vi "RIRetrieval.vi"(0 "Minimization method":u16(ring)=1 items=["LM method", "Simplex Method"], 1 "Extinction Measured Data":T5={"Extinction"=array122x5[610 elements], "Extinction Uncertainty"=array122x5[610 elements], "Size parameters"=array122x5[610 elements], "Number ofSizes"=5.0, "GeometricCrossSection"=[3.1415926535897934e-10, 3.9760782021995823e-10, 4.908738521234053e-10, 5.939573610693203e-10, 7.068583470577035e-10], "WaveLength"=[359.58929, 360.1004, 360.61145, 361.12241, 361.63336, 362.1442, 362.65503, 363.16577, 363.67648, 364.18713, 364.69769, 365.20825, 365.71872, 366.22913, 366.7395, 367.24979, 367.76004, 368.27023, 368.78036, 369.29047, 369.80051, 370.31049, 370.8204, 371.33026, 371.84009, 372.34985, 372.85956, 373.3692, 373.87881, 374.38834, 374.89786, 375.40729, 375.91669, 376.42599, 376.9353, 377.44452, 377.9537, 378.46283, 378.97192, 379.48093, 379.9899, 380.49881, 381.00769, 381.51651, 382.02527, 382.534, 383.04266, 383.55127, 384.05984, 384.56836, 385.07681, 385.58521, 386.09357, 386.6019, 387.11017, 387.61838, 388.12653, 388.63467, 389.14273, 389.65076, 390.15872, 389.65076, 390.15872, 390.66663, 391.17453, 391.68234, 392.19012, 392.69785, 393.20554, 393.71317, 394.22076, 394.7283, 395.23578, 395.74326, 396.25064, 396.758, 397.26532, 397.77258, 398.27979, 398.78696, 399.29407, 399.80115, 400.30817, 400.81516, 401.32211, 401.82901, 402.33585, 402.84265, 403.34943, 403.85614, 404.36282, 404.86945, 405.37604, 405.88257, 406.38907, 406.89554, 407.40195, 407.90833, 408.41464, 408.92093, 409.42715, 409.93335, 410.43951, 410.94562, 411.45169, 411.95773, 412.46371, 412.96964, 413.47556, 413.98141, 414.48724, 414.99301, 415.49875, 416.00446, 416.5101, 417.01572, 417.5213, 418.02682, 418.53235, 419.03778, 419.54321, 420.04858], "Sizes"=[200.0, 225.0, 250.0, 275.0, 300.0], "Concentration (#/cc)"=[]}, 2 "Starting Guess -Real":dbl=1.5, 3 "Approximate Errors":bool, 5 "Graph Refs":T4, 9 "Particle Distribution Data":T6={"SMPS Sizes"=[121.9, 126.3, 131.0, 135.8, 140.7, 145.9, 151.2, 156.8, 162.5, 168.5, 174.7, 181.1, 187.7, 194.6, 201.7, 209.1, 216.7, 224.7, 232.9, 241.4, 250.3, 259.5, 269.0, 278.8, 289.0, 299.6, 310.6, 322.0, 333.8, 346.0, 358.7, 371.8, 385.4, 399.5, 414.2, 429.4, 445.1, 461.4, 478.3, 495.8, 514.0, 532.8, 552.3], "Concentration"=[[0.0, 0.0, 0.0, 0.0, 0.0, 0.0, 0.0, 0.0, 0.0, 0.000594222, 0.0067148, 0.0325883, 0.0950329, 0.181348, 0.216099, 0.185692, 0.101524, 0.0383134, 0.00909043, 0.000780919, 0.0, 0.0, 0.000216077, 0.00198783, 0.0080372, 0.0204479, 0.0283157, 0.0335331, 0.022157, 0.0123005, 0.00284358, 0.000773561, 0.000252233, 0.000229051, 0.000520001, 0.000225684, 0.000138298, 0.000244182, 0.0, 0.0, 0.0, 0.0, 0.0], [0.0, 0.0, 0.0, 0.0, 0.0, 0.0, 0.0, 0.0, 0.0, 0.0, 0.0, 0.0, 0.000816489, 0.00845349, 0.0408459, 0.112602, 0.207837, 0.230678, 0.191195, 0.115028, 0.0385312, 0.00775818, 0.000694285, 0.0, 0.0, 5.45e-05, 0.000573695, 0.00252084, 0.00630844, 0.00962652, 0.0109084, 0.0108076, 0.0029388, 0.00150807, 0.000290999, 2.27e-05, 0.0, 0.0, 0.0, 0.0, 0.0, 0.0, 0.0], [0.0, 0.0, 0.0, 0.0, 0.0, 0.0, 0.0, 0.0, 0.0, 0.0, 0.0, 0.0, 0.0, 0.0, 0.0, 0.0010312, 0.010922, 0.0510087, 0.131879, 0.225192, 0.246535, 0.18825, 0.0982208, 0.0303467, 0.00671228, 0.000607538, 1.36e-05, 0.0, 0.0, 7.85e-05, 0.000394547, 0.00155356, 0.00182002, 0.00285395, 0.00143116, 0.000779854, 0.000340487, 0.0, 0.0, 0.0, 0.0, 0.0, 5.83e-05], [0.0, 0.0, 0.0, 0.0, 0.0, 0.0, 0.0, 0.0, 0.0, 0.0, 0.0, 0.0, 0.0, 0.0, 0.0, 0.0, 0.0, 0.0, 0.00139618, 0.0150043, 0.0584558, 0.144869, 0.242414, 0.233752, 0.174403, 0.0932754, 0.0278801, 0.00466978, 0.000461, 1.86e-05, 0.0, 0.0, 1.87e-05, 0.000141669, 0.000338039, 0.000948904, 0.00124014, 0.000405092, 0.0, 0.000308013, 0.0, 0.0, 0.0], [0.0, 0.0, 0.0, 0.0, 0.0, 0.0, 0.0, 0.0, 0.0, 0.0, 0.0, 0.0, 0.0, 0.0, 0.0, 0.0, 0.0, 0.0, 0.0, 0.0, 0.001984, 0.0181243, 0.0738336, 0.168822, 0.26219, 0.229236, 0.15382, 0.0682415, 0.0199068, 0.0034375, 0.000356967, 1.85e-05, 0.0, 0.0, 7.2e-06, 2.06e-05, 0.0, 0.0, 0.0, 0.0, 0.0, 0.0, 0.0]], "Double Charge Correction Flag"=TRUE}, 11 "Calculate Errors":bool=TRUE, 12 "Restrict to Positive Imaginary Part":bool=TRUE, 13 "Starting Guess - Imag":dbl=0.1, 14 "General Data for RI Retrieval VI":T3={"Min WaveLength Index"=0, "Max WaveLength Index"=121, "Extinction Factor"=FALSE, "Size Parameter Factor"=FALSE, "Size Paramter Offset"=FALSE, "Extinction Factor"=1.0, "Diameter Factor"=1.0, "Diameter Offset"=0.0, "ExtinctionOrAbsorptionOrScattering"=0} {"ExtinctionOrAbsorptionOrScattering" scale=0.0..2.0; "Max WaveLength Index" max=200 step=1; "Min WaveLength Index" max=200 step=1}) -> (4 "Real Part vs wavelength":cluster{dbl[], dbl[]}[](graph)=[{[359.58929, 360.1004, 360.61145, 361.12241, 361.63336, 362.1442, 362.65503, 363.16577, 363.67648, 364.18713, 364.69769, 365.20825, 365.71872, 366.22913, 366.7395, 367.24979, 367.76004, 368.27023, 368.78036, 369.29047, 369.80051, 370.31049, 370.8204, 371.33026, 371.84009, 372.34985, 372.85956, 373.3692, 373.87881, 374.38834, 374.89786, 375.40729, 375.91669, 376.42599, 376.9353, 377.44452, 377.9537, 378.46283, 378.97192, 379.48093, 379.9899, 380.49881, 381.00769, 381.51651, 382.02527, 382.534, 383.04266, 383.55127, 384.05984, 384.56836, 385.07681, 385.58521, 386.09357, 386.6019, 387.11017, 387.61838, 388.12653, 388.63467, 389.14273, 389.65076, 390.15872, 389.65076, 390.15872, 390.66663, 391.17453, 391.68234, 392.19012, 392.69785, 393.20554, 393.71317, 394.22076, 394.7283, 395.23578, 395.74326, 396.25064, 396.758, 397.26532, 397.77258, 398.27979, 398.78696, 399.29407, 399.80115, 400.30817, 400.81516, 401.32211, 401.82901, 402.33585, 402.84265, 403.34943, 403.85614, 404.36282, 404.86945, 405.37604, 405.88257, 406.38907, 406.89554, 407.40195, 407.90833, 408.41464, 408.92093, 409.42715, 409.93335, 410.43951, 410.94562, 411.45169, 411.95773, 412.46371, 412.96964, 413.47556, 413.98141, 414.48724, 414.99301, 415.49875, 416.00446, 416.5101, 417.01572, 417.5213, 418.02682, 418.53235, 419.03778, 419.54321, 420.04858], [1.5396270532046785, 1.538727395001552, 1.534821145001552, 1.5406825036441298, 1.5415669030581922, 1.5455036706363172, 1.5466480798160047, 1.5476615685855357, 1.5472341699038954, 1.5489252824222053, 1.549121510449548, 1.5458964127932977, 1.5447889298831412, 1.5456751603518915, 1.5450364274417363, 1.5443976945315812, 1.5424206728373981, 1.541581134263179, 1.5454557222758747, 1.5423593325053675, 1.537313327256344, 1.5345896334086881, 1.5407291597758752, 1.541564731064938, 1.538654727402829, 1.5370564073955049, 1.5407485765849556, 1.5394119734202825, 1.5341312117015322, 1.536965684357782, 1.5317178816234067, 1.5287030500804377, 1.5274973005687187, 1.5339043898021174, 1.5331876844798522, 1.5293449682628117, 1.5360365600024661, 1.5362565917407474, 1.5274009246264897, 1.5331344623004397, 1.5305994052325689, 1.5268769473468278, 1.5300680369769548, 1.515133306447169, 1.5320916194354501, 1.5417069930468976, 1.537891418400902, 1.5267598266040272, 1.5311928100024632, 1.5343562621509004, 1.5248573607837126, 1.5298715514575405, 1.5194143981372292, 1.521543304387229, 1.5345590919886996, 1.5370029396449496, 1.5382092995082304, 1.5201217598353787, 1.533493494454519, 1.5250244087611615, 1.528523096505302, 1.5305934090053022, 1.5374183601771767, 1.523488001290457, 1.51958495563616, 1.5280126900111597, 1.5125830025111582, 1.5290344185267832, 1.5172637886439704, 1.5226925987635989, 1.5252196068202393, 1.5269847435389892, 1.5132711822425255, 1.5168063384925254, 1.5125790435706503, 1.5172769195472116, 1.5246480590735807, 1.5129183012877858, 1.517646694842472, 1.5133032042418861, 1.5151971251403236, 1.5191888243590723, 1.5131286436950102, 1.5062460143004799, 1.5115656859313376, 1.5106379515563368, 1.512958508196962, 1.511806774798524, 1.5120249754821184, 1.5104307372008678, 1.5129768378173223, 1.5112502867614142, 1.5110824400817269, 1.5072253233825075, 1.502771015826355, 1.5042590529357298, 1.502026997271666, 1.497705746356139, 1.4951637179290151, 1.496234217349181, 1.492047072116026, 1.4983118111525868, 1.4949415547286367, 1.4929246861373284, 1.4926866275702815, 1.490306308928619, 1.4843443567191468, 1.4885330349837649, 1.493107185426842, 1.4893548203145373, 1.4812372971211785, 1.4947460747395862, 1.4976160240804064, 1.4870664024983753, 1.4926434076463098, 1.4957490176593176, 1.4934942263995516, 1.4954207820330967, 1.4921062869464272, 1.493986455861222, 1.4937534350787511, 1.4779602021609655]}, {[359.58929, 359.58929, 359.58929, 360.1004, 360.1004, 360.1004, 360.61145, 360.61145, 360.61145, 361.12241, 361.12241, 361.12241, 361.63336, 361.63336, 361.63336, 362.1442, 362.1442, 362.1442, 362.65503, 362.65503, 362.65503, 363.16577, 363.16577, 363.16577, 363.67648, 363.67648, 363.67648, 364.18713, 364.18713, 364.18713, 364.69769, 364.69769, 364.69769, 365.20825, 365.20825, 365.20825, 365.71872, 365.71872, 365.71872, 366.22913, 366.22913, 366.22913, 366.7395, 366.7395, 366.7395, 367.24979, 367.24979, 367.24979, 367.76004, 367.76004, 367.76004, 368.27023, 368.27023, 368.27023, 368.78036, 368.78036, 368.78036, 369.29047, 369.29047, 369.29047, 369.80051, 369.80051, 369.80051, 370.31049, 370.31049, 370.31049, 370.8204, 370.8204, 370.8204, 371.33026, 371.33026, 371.33026, 371.84009, 371.84009, 371.84009, 372.34985, 372.34985, 372.34985, 372.85956, 372.85956, 372.85956, 373.3692, 373.3692, 373.3692, 373.87881, 373.87881, 373.87881, 374.38834, 374.38834, 374.38834, 374.89786, 374.89786, 374.89786, 375.40729, 375.40729, 375.40729, 375.91669, 375.91669, 375.91669, 376.42599, 376.42599, 376.42599, 376.9353, 376.9353, 376.9353, 377.44452, 377.44452, 377.44452, 377.9537, 377.9537, 377.9537, 378.46283, 378.46283, 378.46283, 378.97192, 378.97192, 378.97192, 379.48093, 379.48093, 379.48093, 379.9899, 379.9899, 379.9899, 380.49881, 380.49881, 380.49881, 381.00769, 381.00769, 381.00769, 381.51651, 381.51651, 381.51651, 382.02527, 382.02527, 382.02527, 382.534, 382.534, 382.534, 383.04266, 383.04266, 383.04266, 383.55127, 383.55127, 383.55127, 384.05984, 384.05984, 384.05984, 384.56836, 384.56836, 384.56836, 385.07681, 385.07681, 385.07681, 385.58521, 385.58521, 385.58521, 386.09357, 386.09357, 386.09357, 386.6019, 386.6019, 386.6019, 387.11017, 387.11017, 387.11017, 387.61838, 387.61838, 387.61838, 388.12653, 388.12653, 388.12653, 388.63467, 388.63467, 388.63467, 389.14273, 389.14273, 389.14273, 389.65076, 389.65076, 389.65076, 390.15872, 390.15872, 390.15872, 389.65076, 389.65076, 389.65076, 390.15872, 390.15872, 390.15872, 390.66663, 390.66663, 390.66663, 391.17453, 391.17453, 391.17453, 391.68234, 391.68234, 391.68234, 392.19012, 392.19012, 392.19012, 392.69785, 392.69785, 392.69785, 393.20554, 393.20554, 393.20554, 393.71317, 393.71317, 393.71317, 394.22076, 394.22076, 394.22076, 394.7283, 394.7283, 394.7283, 395.23578, 395.23578, 395.23578, 395.74326, 395.74326, 395.74326, 396.25064, 396.25064, 396.25064, 396.758, 396.758, 396.758, 397.26532, 397.26532, 397.26532, 397.77258, 397.77258, 397.77258, 398.27979, 398.27979, 398.27979, 398.78696, 398.78696, 398.78696, 399.29407, 399.29407, 399.29407, 399.80115, 399.80115, 399.80115, 400.30817, 400.30817, 400.30817, 400.81516, 400.81516, 400.81516, 401.32211, 401.32211, 401.32211, 401.82901, 401.82901, 401.82901, 402.33585, 402.33585, 402.33585, 402.84265, 402.84265, 402.84265, 403.34943, 403.34943, 403.34943, 403.85614, 403.85614, 403.85614, 404.36282, 404.36282, 404.36282, 404.86945, 404.86945, 404.86945, 405.37604, 405.37604, 405.37604, 405.88257, 405.88257, 405.88257, 406.38907, 406.38907, 406.38907, 406.89554, 406.89554, 406.89554, 407.40195, 407.40195, 407.40195, 407.90833, 407.90833, 407.90833, 408.41464, 408.41464, 408.41464, 408.92093, 408.92093, 408.92093, 409.42715, 409.42715, 409.42715, 409.93335, 409.93335, 409.93335, 410.43951, 410.43951, 410.43951, 410.94562, 410.94562, 410.94562, 411.45169, 411.45169, 411.45169, 411.95773, 411.95773, 411.95773, 412.46371, 412.46371, 412.46371, 412.96964, 412.96964, 412.96964, 413.47556, 413.47556, 413.47556, 413.98141, 413.98141, 413.98141, 414.48724, 414.48724, 414.48724, 414.99301, 414.99301, 414.99301, 415.49875, 415.49875, 415.49875, 416.00446, 416.00446, 416.00446, 416.5101, 416.5101, 416.5101, 417.01572, 417.01572, 417.01572, 417.5213, 417.5213, 417.5213, 418.02682, 418.02682, 418.02682, 418.53235, 418.53235, 418.53235, 419.03778, 419.03778, 419.03778, 419.54321, 419.54321, 419.54321, 420.04858, 420.04858, 420.04858], [nan, 1.5396270532046785, 1.5396270532046785, nan, 1.538727395001552, 1.538727395001552, nan, 1.534821145001552, 1.534821145001552, nan, 1.5406825036441298, 1.5406825036441298, nan, 1.5415669030581922, 1.5415669030581922, nan, 1.5455036706363172, 1.5455036706363172, nan, 1.5466480798160047, 1.5466480798160047, nan, 1.5476615685855357, 1.5476615685855357, nan, 1.5472341699038954, 1.5472341699038954, nan, 1.5489252824222053, 1.5489252824222053, nan, 1.549121510449548, 1.549121510449548, nan, 1.5458964127932977, 1.5458964127932977, nan, 1.5447889298831412, 1.5447889298831412, nan, 1.5456751603518915, 1.5456751603518915, nan, 1.5450364274417363, 1.5450364274417363, nan, 1.5443976945315812, 1.5443976945315812, nan, 1.5424206728373981, 1.5424206728373981, nan, 1.541581134263179, 1.541581134263179, nan, 1.5454557222758747, 1.5454557222758747, nan, 1.5423593325053675, 1.5423593325053675, nan, 1.537313327256344, 1.537313327256344, nan, 1.5345896334086881, 1.5345896334086881, nan, 1.5407291597758752, 1.5407291597758752, nan, 1.541564731064938, 1.541564731064938, nan, 1.538654727402829, 1.538654727402829, nan, 1.5370564073955049, 1.5370564073955049, nan, 1.5407485765849556, 1.5407485765849556, nan, 1.5394119734202825, 1.5394119734202825, nan, 1.5341312117015322, 1.5341312117015322, nan, 1.536965684357782, 1.536965684357782, nan, 1.5317178816234067, 1.5317178816234067, nan, 1.5287030500804377, 1.5287030500804377, nan, 1.5274973005687187, 1.5274973005687187, nan, 1.5339043898021174, 1.5339043898021174, nan, 1.5331876844798522, 1.5331876844798522, nan, 1.5293449682628117, 1.5293449682628117, nan, 1.5360365600024661, 1.5360365600024661, nan, 1.5362565917407474, 1.5362565917407474, nan, 1.5274009246264897, 1.5274009246264897, nan, 1.5331344623004397, 1.5331344623004397, nan, 1.5305994052325689, 1.5305994052325689, nan, 1.5268769473468278, 1.5268769473468278, nan, 1.5300680369769548, 1.5300680369769548, nan, 1.515133306447169, 1.515133306447169, nan, 1.5320916194354501, 1.5320916194354501, nan, 1.5417069930468976, 1.5417069930468976, nan, 1.537891418400902, 1.537891418400902, nan, 1.5267598266040272, 1.5267598266040272, nan, 1.5311928100024632, 1.5311928100024632, nan, 1.5343562621509004, 1.5343562621509004, nan, 1.5248573607837126, 1.5248573607837126, nan, 1.5298715514575405, 1.5298715514575405, nan, 1.5194143981372292, 1.5194143981372292, nan, 1.521543304387229, 1.521543304387229, nan, 1.5345590919886996, 1.5345590919886996, nan, 1.5370029396449496, 1.5370029396449496, nan, 1.5382092995082304, 1.5382092995082304, nan, 1.5201217598353787, 1.5201217598353787, nan, 1.533493494454519, 1.533493494454519, nan, 1.5250244087611615, 1.5250244087611615, nan, 1.528523096505302, 1.528523096505302, nan, 1.5305934090053022, 1.5305934090053022, nan, 1.5374183601771767, 1.5374183601771767, nan, 1.523488001290457, 1.523488001290457, nan, 1.51958495563616, 1.51958495563616, nan, 1.5280126900111597, 1.5280126900111597, nan, 1.5125830025111582, 1.5125830025111582, nan, 1.5290344185267832, 1.5290344185267832, nan, 1.5172637886439704, 1.5172637886439704, nan, 1.5226925987635989, 1.5226925987635989, nan, 1.5252196068202393, 1.5252196068202393, nan, 1.5269847435389892, 1.5269847435389892, nan, 1.5132711822425255, 1.5132711822425255, nan, 1.5168063384925254, 1.5168063384925254, nan, 1.5125790435706503, 1.5125790435706503, nan, 1.5172769195472116, 1.5172769195472116, nan, 1.5246480590735807, 1.5246480590735807, nan, 1.5129183012877858, 1.5129183012877858, nan, 1.517646694842472, 1.517646694842472, nan, 1.5133032042418861, 1.5133032042418861, nan, 1.5151971251403236, 1.5151971251403236, nan, 1.5191888243590723, 1.5191888243590723, nan, 1.5131286436950102, 1.5131286436950102, nan, 1.5062460143004799, 1.5062460143004799, nan, 1.5115656859313376, 1.5115656859313376, nan, 1.5106379515563368, 1.5106379515563368, nan, 1.512958508196962, 1.512958508196962, nan, 1.511806774798524, 1.511806774798524, nan, 1.5120249754821184, 1.5120249754821184, nan, 1.5104307372008678, 1.5104307372008678, nan, 1.5129768378173223, 1.5129768378173223, nan, 1.5112502867614142, 1.5112502867614142, nan, 1.5110824400817269, 1.5110824400817269, nan, 1.5072253233825075, 1.5072253233825075, nan, 1.502771015826355, 1.502771015826355, nan, 1.5042590529357298, 1.5042590529357298, nan, 1.502026997271666, 1.502026997271666, nan, 1.497705746356139, 1.497705746356139, nan, 1.4951637179290151, 1.4951637179290151, nan, 1.496234217349181, 1.496234217349181, nan, 1.492047072116026, 1.492047072116026, nan, 1.4983118111525868, 1.4983118111525868, nan, 1.4949415547286367, 1.4949415547286367, nan, 1.4929246861373284, 1.4929246861373284, nan, 1.4926866275702815, 1.4926866275702815, nan, 1.490306308928619, 1.490306308928619, nan, 1.4843443567191468, 1.4843443567191468, nan, 1.4885330349837649, 1.4885330349837649, nan, 1.493107185426842, 1.493107185426842, nan, 1.4893548203145373, 1.4893548203145373, nan, 1.4812372971211785, 1.4812372971211785, nan, 1.4947460747395862, 1.4947460747395862, nan, 1.4976160240804064, 1.4976160240804064, nan, 1.4870664024983753, 1.4870664024983753, nan, 1.4926434076463098, 1.4926434076463098, nan, 1.4957490176593176, 1.4957490176593176, nan, 1.4934942263995516, 1.4934942263995516, nan, 1.4954207820330967, 1.4954207820330967, nan, 1.4921062869464272, 1.4921062869464272, nan, 1.493986455861222, 1.493986455861222, nan, 1.4937534350787511, 1.4937534350787511, nan, 1.4779602021609655, 1.4779602021609655]}, {[359.58929, 360.1004, 360.61145, 361.12241, 361.63336, 362.1442, 362.65503, 363.16577, 363.67648, 364.18713, 364.69769, 365.20825, 365.71872, 366.22913, 366.7395, 367.24979, 367.76004, 368.27023, 368.78036, 369.29047, 369.80051, 370.31049, 370.8204, 371.33026, 371.84009, 372.34985, 372.85956, 373.3692, 373.87881, 374.38834, 374.89786, 375.40729, 375.91669, 376.42599, 376.9353, 377.44452, 377.9537, 378.46283, 378.97192, 379.48093, 379.9899, 380.49881, 381.00769, 381.51651, 382.02527, 382.534, 383.04266, 383.55127, 384.05984, 384.56836, 385.07681, 385.58521, 386.09357, 386.6019, 387.11017, 387.61838, 388.12653, 388.63467, 389.14273, 389.65076, 390.15872, 389.65076, 390.15872, 390.66663, 391.17453, 391.68234, 392.19012, 392.69785, 393.20554, 393.71317, 394.22076, 394.7283, 395.23578, 395.74326, 396.25064, 396.758, 397.26532, 397.77258, 398.27979, 398.78696, 399.29407, 399.80115, 400.30817, 400.81516, 401.32211, 401.82901, 402.33585, 402.84265, 403.34943, 403.85614, 404.36282, 404.86945, 405.37604, 405.88257, 406.38907, 406.89554, 407.40195, 407.90833, 408.41464, 408.92093, 409.42715, 409.93335, 410.43951, 410.94562, 411.45169, 411.95773, 412.46371, 412.96964, 413.47556, 413.98141, 414.48724, 414.99301, 415.49875, 416.00446, 416.5101, 417.01572, 417.5213, 418.02682, 418.53235, 419.03778, 419.54321, 420.04858], [1.5396270532046785, 1.538727395001552, 1.534821145001552, 1.5406825036441298, 1.5415669030581922, 1.5455036706363172, 1.5466480798160047, 1.5476615685855357, 1.5472341699038954, 1.5489252824222053, 1.549121510449548, 1.5458964127932977, 1.5447889298831412, 1.5456751603518915, 1.5450364274417363, 1.5443976945315812, 1.5424206728373981, 1.541581134263179, 1.5454557222758747, 1.5423593325053675, 1.537313327256344, 1.5345896334086881, 1.5407291597758752, 1.541564731064938, 1.538654727402829, 1.5370564073955049, 1.5407485765849556, 1.5394119734202825, 1.5341312117015322, 1.536965684357782, 1.5317178816234067, 1.5287030500804377, 1.5274973005687187, 1.5339043898021174, 1.5331876844798522, 1.5293449682628117, 1.5360365600024661, 1.5362565917407474, 1.5274009246264897, 1.5331344623004397, 1.5305994052325689, 1.5268769473468278, 1.5300680369769548, 1.515133306447169, 1.5320916194354501, 1.5417069930468976, 1.537891418400902, 1.5267598266040272, 1.5311928100024632, 1.5343562621509004, 1.5248573607837126, 1.5298715514575405, 1.5194143981372292, 1.521543304387229, 1.5345590919886996, 1.5370029396449496, 1.5382092995082304, 1.5201217598353787, 1.533493494454519, 1.5250244087611615, 1.528523096505302, 1.5305934090053022, 1.5374183601771767, 1.523488001290457, 1.51958495563616, 1.5280126900111597, 1.5125830025111582, 1.5290344185267832, 1.5172637886439704, 1.5226925987635989, 1.5252196068202393, 1.5269847435389892, 1.5132711822425255, 1.5168063384925254, 1.5125790435706503, 1.5172769195472116, 1.5246480590735807, 1.5129183012877858, 1.517646694842472, 1.5133032042418861, 1.5151971251403236, 1.5191888243590723, 1.5131286436950102, 1.5062460143004799, 1.5115656859313376, 1.5106379515563368, 1.512958508196962, 1.511806774798524, 1.5120249754821184, 1.5104307372008678, 1.5129768378173223, 1.5112502867614142, 1.5110824400817269, 1.5072253233825075, 1.502771015826355, 1.5042590529357298, 1.502026997271666, 1.497705746356139, 1.4951637179290151, 1.496234217349181, 1.492047072116026, 1.4983118111525868, 1.4949415547286367, 1.4929246861373284, 1.4926866275702815, 1.490306308928619, 1.4843443567191468, 1.4885330349837649, 1.493107185426842, 1.4893548203145373, 1.4812372971211785, 1.4947460747395862, 1.4976160240804064, 1.4870664024983753, 1.4926434076463098, 1.4957490176593176, 1.4934942263995516, 1.4954207820330967, 1.4921062869464272, 1.493986455861222, 1.4937534350787511, 1.4779602021609655]}], 6 "RI results":T2={"Real RI"=[1.5396270532046785, 1.538727395001552, 1.534821145001552, 1.5406825036441298, 1.5415669030581922, 1.5455036706363172, 1.5466480798160047, 1.5476615685855357, 1.5472341699038954, 1.5489252824222053, 1.549121510449548, 1.5458964127932977, 1.5447889298831412, 1.5456751603518915, 1.5450364274417363, 1.5443976945315812, 1.5424206728373981, 1.541581134263179, 1.5454557222758747, 1.5423593325053675, 1.537313327256344, 1.5345896334086881, 1.5407291597758752, 1.541564731064938, 1.538654727402829, 1.5370564073955049, 1.5407485765849556, 1.5394119734202825, 1.5341312117015322, 1.536965684357782, 1.5317178816234067, 1.5287030500804377, 1.5274973005687187, 1.5339043898021174, 1.5331876844798522, 1.5293449682628117, 1.5360365600024661, 1.5362565917407474, 1.5274009246264897, 1.5331344623004397, 1.5305994052325689, 1.5268769473468278, 1.5300680369769548, 1.515133306447169, 1.5320916194354501, 1.5417069930468976, 1.537891418400902, 1.5267598266040272, 1.5311928100024632, 1.5343562621509004, 1.5248573607837126, 1.5298715514575405, 1.5194143981372292, 1.521543304387229, 1.5345590919886996, 1.5370029396449496, 1.5382092995082304, 1.5201217598353787, 1.533493494454519, 1.5250244087611615, 1.528523096505302, 1.5305934090053022, 1.5374183601771767, 1.523488001290457, 1.51958495563616, 1.5280126900111597, 1.5125830025111582, 1.5290344185267832, 1.5172637886439704, 1.5226925987635989, 1.5252196068202393, 1.5269847435389892, 1.5132711822425255, 1.5168063384925254, 1.5125790435706503, 1.5172769195472116, 1.5246480590735807, 1.5129183012877858, 1.517646694842472, 1.5133032042418861, 1.5151971251403236, 1.5191888243590723, 1.5131286436950102, 1.5062460143004799, 1.5115656859313376, 1.5106379515563368, 1.512958508196962, 1.511806774798524, 1.5120249754821184, 1.5104307372008678, 1.5129768378173223, 1.5112502867614142, 1.5110824400817269, 1.5072253233825075, 1.502771015826355, 1.5042590529357298, 1.502026997271666, 1.497705746356139, 1.4951637179290151, 1.496234217349181, 1.492047072116026, 1.4983118111525868, 1.4949415547286367, 1.4929246861373284, 1.4926866275702815, 1.490306308928619, 1.4843443567191468, 1.4885330349837649, 1.493107185426842, 1.4893548203145373, 1.4812372971211785, 1.4947460747395862, 1.4976160240804064, 1.4870664024983753, 1.4926434076463098, 1.4957490176593176, 1.4934942263995516, 1.4954207820330967, 1.4921062869464272, 1.493986455861222, 1.4937534350787511, 1.4779602021609655], "Imaginary RI"=[0.014012220551121871, 0.0, 0.0, 0.005994377136230469, 0.0, 0.0, 0.004224395751953125, 0.0, 0.0038824844360351553, 0.0, 0.0, 0.0, 0.0, 0.0, 0.0, 0.0, 0.0, 0.0, 0.00019025802612304666, 0.0, 0.0, 0.0, 0.002421417236328125, 0.0, 0.0006414413452148437, 0.007469778060913087, 0.0, 0.0, 0.0, 0.0, 0.0, 0.0, 0.0, 0.0, 0.0156949234008789, 0.026187481880187977, 0.023743436932563776, 0.028988721966743465, 0.02145364582538604, 0.011232057213783255, 0.024074302315711966, 0.0, 0.005289626121520995, 0.025243592262268064, 0.0072573709487915045, 0.0, 0.002139425277709961, 0.0, 0.0, 0.0, 0.0, 0.0, 0.0, 0.0, 0.005034195780754091, 0.0, 0.0, 0.011182727813720702, 0.014443035125732414, 0.03869737625122069, 0.010358257293701132, 0.0, 0.0, 0.0, 0.0, 0.0, 0.0, 0.0, 0.0, 0.0, 0.0, 0.0, 0.010822300016880039, 0.0, 0.0, 0.0, 0.0, 0.0, 0.0, 0.0, 0.0, 0.0, 0.0, 0.0, 0.0, 0.0, 0.0, 0.0, 0.0, 0.0, 0.0, 0.0, 0.001330413818359375, 0.0, 0.005959672927856445, 0.0, 0.0, 0.007199201583862303, 0.015323598384857178, 0.006805078983306886, 0.015063683986663825, 0.0027363955974578887, 0.012695561647415168, 0.014204474687576312, 0.005719540715217604, 0.01737168252468111, 0.02141170442104342, 0.017217719554901152, 0.01012599721550945, 0.01238225713372234, 0.02997728124260906, 0.0, 0.008400363922119142, 0.01761590957641602, 0.010009559690952293, 0.008900764733552925, 0.014991348534822459, 0.009456551820039742, 0.018010605126619325, 0.011810782700777043, 0.00289439991116523, 0.023103605061769474], "Std Imaginary RI"=[0.0, 0.0, 0.0, 0.0, 0.0, 0.0, 0.0, 0.0, 0.0, 0.0, 0.0, 0.0, 0.0, 0.0, 0.0, 0.0, 0.0, 0.0, 0.0, 0.0, 0.0, 0.0, 0.0, 0.0, 0.0, 0.0, 0.0, 0.0, 0.0, 0.0, 0.0, 0.0, 0.0, 0.0, 0.0, 0.0, 0.0, 0.0, 0.0, 0.0, 0.0, 0.0, 0.0, 0.0, 0.0, 0.0, 0.0, 0.0, 0.0, 0.0, 0.0, 0.0, 0.0, 0.0, 0.0, 0.0, 0.0, 0.0, 0.0, 0.0, 0.0, 0.0, 0.0, 0.0, 0.0, 0.0, 0.0, 0.0, 0.0, 0.0, 0.0, 0.0, 0.0, 0.0, 0.0, 0.0, 0.0, 0.0, 0.0, 0.0, 0.0, 0.0, 0.0, 0.0, 0.0, 0.0, 0.0, 0.0, 0.0, 0.0, 0.0, 0.0, 0.0, 0.0, 0.0, 0.0, 0.0, 0.0, 0.0, 0.0, 0.0, 0.0, 0.0, 0.0, 0.0, 0.0, 0.0, 0.0, 0.0, 0.0, 0.0, 0.0, 0.0, 0.0, 0.0, 0.0, 0.0, 0.0, 0.0, 0.0, 0.0, 0.0], "Std Real RI"=[0.0, 0.0, 0.0, 0.0, 0.0, 0.0, 0.0, 0.0, 0.0, 0.0, 0.0, 0.0, 0.0, 0.0, 0.0, 0.0, 0.0, 0.0, 0.0, 0.0, 0.0, 0.0, 0.0, 0.0, 0.0, 0.0, 0.0, 0.0, 0.0, 0.0, 0.0, 0.0, 0.0, 0.0, 0.0, 0.0, 0.0, 0.0, 0.0, 0.0, 0.0, 0.0, 0.0, 0.0, 0.0, 0.0, 0.0, 0.0, 0.0, 0.0, 0.0, 0.0, 0.0, 0.0, 0.0, 0.0, 0.0, 0.0, 0.0, 0.0, 0.0, 0.0, 0.0, 0.0, 0.0, 0.0, 0.0, 0.0, 0.0, 0.0, 0.0, 0.0, 0.0, 0.0, 0.0, 0.0, 0.0, 0.0, 0.0, 0.0, 0.0, 0.0, 0.0, 0.0, 0.0, 0.0, 0.0, 0.0, 0.0, 0.0, 0.0, 0.0, 0.0, 0.0, 0.0, 0.0, 0.0, 0.0, 0.0, 0.0, 0.0, 0.0, 0.0, 0.0, 0.0, 0.0, 0.0, 0.0, 0.0, 0.0, 0.0, 0.0, 0.0, 0.0, 0.0, 0.0, 0.0, 0.0, 0.0, 0.0, 0.0, 0.0], "Wavelength"=[359.58929, 360.1004, 360.61145, 361.12241, 361.63336, 362.1442, 362.65503, 363.16577, 363.67648, 364.18713, 364.69769, 365.20825, 365.71872, 366.22913, 366.7395, 367.24979, 367.76004, 368.27023, 368.78036, 369.29047, 369.80051, 370.31049, 370.8204, 371.33026, 371.84009, 372.34985, 372.85956, 373.3692, 373.87881, 374.38834, 374.89786, 375.40729, 375.91669, 376.42599, 376.9353, 377.44452, 377.9537, 378.46283, 378.97192, 379.48093, 379.9899, 380.49881, 381.00769, 381.51651, 382.02527, 382.534, 383.04266, 383.55127, 384.05984, 384.56836, 385.07681, 385.58521, 386.09357, 386.6019, 387.11017, 387.61838, 388.12653, 388.63467, 389.14273, 389.65076, 390.15872, 389.65076, 390.15872, 390.66663, 391.17453, 391.68234, 392.19012, 392.69785, 393.20554, 393.71317, 394.22076, 394.7283, 395.23578, 395.74326, 396.25064, 396.758, 397.26532, 397.77258, 398.27979, 398.78696, 399.29407, 399.80115, 400.30817, 400.81516, 401.32211, 401.82901, 402.33585, 402.84265, 403.34943, 403.85614, 404.36282, 404.86945, 405.37604, 405.88257, 406.38907, 406.89554, 407.40195, 407.90833, 408.41464, 408.92093, 409.42715, 409.93335, 410.43951, 410.94562, 411.45169, 411.95773, 412.46371, 412.96964, 413.47556, 413.98141, 414.48724, 414.99301, 415.49875, 416.00446, 416.5101, 417.01572, 417.5213, 418.02682, 418.53235, 419.03778, 419.54321, 420.04858], "Residue"=[], "Extinction Factor"=[], "Diameter Factor"=[], "Diameter Offset"=[], "Best fit result"=[], "Normalized Residuals"=[]}, 10 "Imaginary Part vs wavelength":cluster{dbl[], dbl[]}[](graph)=[{[359.58929, 360.1004, 360.61145, 361.12241, 361.63336, 362.1442, 362.65503, 363.16577, 363.67648, 364.18713, 364.69769, 365.20825, 365.71872, 366.22913, 366.7395, 367.24979, 367.76004, 368.27023, 368.78036, 369.29047, 369.80051, 370.31049, 370.8204, 371.33026, 371.84009, 372.34985, 372.85956, 373.3692, 373.87881, 374.38834, 374.89786, 375.40729, 375.91669, 376.42599, 376.9353, 377.44452, 377.9537, 378.46283, 378.97192, 379.48093, 379.9899, 380.49881, 381.00769, 381.51651, 382.02527, 382.534, 383.04266, 383.55127, 384.05984, 384.56836, 385.07681, 385.58521, 386.09357, 386.6019, 387.11017, 387.61838, 388.12653, 388.63467, 389.14273, 389.65076, 390.15872, 389.65076, 390.15872, 390.66663, 391.17453, 391.68234, 392.19012, 392.69785, 393.20554, 393.71317, 394.22076, 394.7283, 395.23578, 395.74326, 396.25064, 396.758, 397.26532, 397.77258, 398.27979, 398.78696, 399.29407, 399.80115, 400.30817, 400.81516, 401.32211, 401.82901, 402.33585, 402.84265, 403.34943, 403.85614, 404.36282, 404.86945, 405.37604, 405.88257, 406.38907, 406.89554, 407.40195, 407.90833, 408.41464, 408.92093, 409.42715, 409.93335, 410.43951, 410.94562, 411.45169, 411.95773, 412.46371, 412.96964, 413.47556, 413.98141, 414.48724, 414.99301, 415.49875, 416.00446, 416.5101, 417.01572, 417.5213, 418.02682, 418.53235, 419.03778, 419.54321, 420.04858], [0.014012220551121871, 0.0, 0.0, 0.005994377136230469, 0.0, 0.0, 0.004224395751953125, 0.0, 0.0038824844360351553, 0.0, 0.0, 0.0, 0.0, 0.0, 0.0, 0.0, 0.0, 0.0, 0.00019025802612304666, 0.0, 0.0, 0.0, 0.002421417236328125, 0.0, 0.0006414413452148437, 0.007469778060913087, 0.0, 0.0, 0.0, 0.0, 0.0, 0.0, 0.0, 0.0, 0.0156949234008789, 0.026187481880187977, 0.023743436932563776, 0.028988721966743465, 0.02145364582538604, 0.011232057213783255, 0.024074302315711966, 0.0, 0.005289626121520995, 0.025243592262268064, 0.0072573709487915045, 0.0, 0.002139425277709961, 0.0, 0.0, 0.0, 0.0, 0.0, 0.0, 0.0, 0.005034195780754091, 0.0, 0.0, 0.011182727813720702, 0.014443035125732414, 0.03869737625122069, 0.010358257293701132, 0.0, 0.0, 0.0, 0.0, 0.0, 0.0, 0.0, 0.0, 0.0, 0.0, 0.0, 0.010822300016880039, 0.0, 0.0, 0.0, 0.0, 0.0, 0.0, 0.0, 0.0, 0.0, 0.0, 0.0, 0.0, 0.0, 0.0, 0.0, 0.0, 0.0, 0.0, 0.0, 0.001330413818359375, 0.0, 0.005959672927856445, 0.0, 0.0, 0.007199201583862303, 0.015323598384857178, 0.006805078983306886, 0.015063683986663825, 0.0027363955974578887, 0.012695561647415168, 0.014204474687576312, 0.005719540715217604, 0.01737168252468111, 0.02141170442104342, 0.017217719554901152, 0.01012599721550945, 0.01238225713372234, 0.02997728124260906, 0.0, 0.008400363922119142, 0.01761590957641602, 0.010009559690952293, 0.008900764733552925, 0.014991348534822459, 0.009456551820039742, 0.018010605126619325, 0.011810782700777043, 0.00289439991116523, 0.023103605061769474]}, {[359.58929, 359.58929, 359.58929, 360.1004, 360.1004, 360.1004, 360.61145, 360.61145, 360.61145, 361.12241, 361.12241, 361.12241, 361.63336, 361.63336, 361.63336, 362.1442, 362.1442, 362.1442, 362.65503, 362.65503, 362.65503, 363.16577, 363.16577, 363.16577, 363.67648, 363.67648, 363.67648, 364.18713, 364.18713, 364.18713, 364.69769, 364.69769, 364.69769, 365.20825, 365.20825, 365.20825, 365.71872, 365.71872, 365.71872, 366.22913, 366.22913, 366.22913, 366.7395, 366.7395, 366.7395, 367.24979, 367.24979, 367.24979, 367.76004, 367.76004, 367.76004, 368.27023, 368.27023, 368.27023, 368.78036, 368.78036, 368.78036, 369.29047, 369.29047, 369.29047, 369.80051, 369.80051, 369.80051, 370.31049, 370.31049, 370.31049, 370.8204, 370.8204, 370.8204, 371.33026, 371.33026, 371.33026, 371.84009, 371.84009, 371.84009, 372.34985, 372.34985, 372.34985, 372.85956, 372.85956, 372.85956, 373.3692, 373.3692, 373.3692, 373.87881, 373.87881, 373.87881, 374.38834, 374.38834, 374.38834, 374.89786, 374.89786, 374.89786, 375.40729, 375.40729, 375.40729, 375.91669, 375.91669, 375.91669, 376.42599, 376.42599, 376.42599, 376.9353, 376.9353, 376.9353, 377.44452, 377.44452, 377.44452, 377.9537, 377.9537, 377.9537, 378.46283, 378.46283, 378.46283, 378.97192, 378.97192, 378.97192, 379.48093, 379.48093, 379.48093, 379.9899, 379.9899, 379.9899, 380.49881, 380.49881, 380.49881, 381.00769, 381.00769, 381.00769, 381.51651, 381.51651, 381.51651, 382.02527, 382.02527, 382.02527, 382.534, 382.534, 382.534, 383.04266, 383.04266, 383.04266, 383.55127, 383.55127, 383.55127, 384.05984, 384.05984, 384.05984, 384.56836, 384.56836, 384.56836, 385.07681, 385.07681, 385.07681, 385.58521, 385.58521, 385.58521, 386.09357, 386.09357, 386.09357, 386.6019, 386.6019, 386.6019, 387.11017, 387.11017, 387.11017, 387.61838, 387.61838, 387.61838, 388.12653, 388.12653, 388.12653, 388.63467, 388.63467, 388.63467, 389.14273, 389.14273, 389.14273, 389.65076, 389.65076, 389.65076, 390.15872, 390.15872, 390.15872, 389.65076, 389.65076, 389.65076, 390.15872, 390.15872, 390.15872, 390.66663, 390.66663, 390.66663, 391.17453, 391.17453, 391.17453, 391.68234, 391.68234, 391.68234, 392.19012, 392.19012, 392.19012, 392.69785, 392.69785, 392.69785, 393.20554, 393.20554, 393.20554, 393.71317, 393.71317, 393.71317, 394.22076, 394.22076, 394.22076, 394.7283, 394.7283, 394.7283, 395.23578, 395.23578, 395.23578, 395.74326, 395.74326, 395.74326, 396.25064, 396.25064, 396.25064, 396.758, 396.758, 396.758, 397.26532, 397.26532, 397.26532, 397.77258, 397.77258, 397.77258, 398.27979, 398.27979, 398.27979, 398.78696, 398.78696, 398.78696, 399.29407, 399.29407, 399.29407, 399.80115, 399.80115, 399.80115, 400.30817, 400.30817, 400.30817, 400.81516, 400.81516, 400.81516, 401.32211, 401.32211, 401.32211, 401.82901, 401.82901, 401.82901, 402.33585, 402.33585, 402.33585, 402.84265, 402.84265, 402.84265, 403.34943, 403.34943, 403.34943, 403.85614, 403.85614, 403.85614, 404.36282, 404.36282, 404.36282, 404.86945, 404.86945, 404.86945, 405.37604, 405.37604, 405.37604, 405.88257, 405.88257, 405.88257, 406.38907, 406.38907, 406.38907, 406.89554, 406.89554, 406.89554, 407.40195, 407.40195, 407.40195, 407.90833, 407.90833, 407.90833, 408.41464, 408.41464, 408.41464, 408.92093, 408.92093, 408.92093, 409.42715, 409.42715, 409.42715, 409.93335, 409.93335, 409.93335, 410.43951, 410.43951, 410.43951, 410.94562, 410.94562, 410.94562, 411.45169, 411.45169, 411.45169, 411.95773, 411.95773, 411.95773, 412.46371, 412.46371, 412.46371, 412.96964, 412.96964, 412.96964, 413.47556, 413.47556, 413.47556, 413.98141, 413.98141, 413.98141, 414.48724, 414.48724, 414.48724, 414.99301, 414.99301, 414.99301, 415.49875, 415.49875, 415.49875, 416.00446, 416.00446, 416.00446, 416.5101, 416.5101, 416.5101, 417.01572, 417.01572, 417.01572, 417.5213, 417.5213, 417.5213, 418.02682, 418.02682, 418.02682, 418.53235, 418.53235, 418.53235, 419.03778, 419.03778, 419.03778, 419.54321, 419.54321, 419.54321, 420.04858, 420.04858, 420.04858], [nan, 0.014012220551121871, 0.014012220551121871, nan, 0.0, 0.0, nan, 0.0, 0.0, nan, 0.005994377136230469, 0.005994377136230469, nan, 0.0, 0.0, nan, 0.0, 0.0, nan, 0.004224395751953125, 0.004224395751953125, nan, 0.0, 0.0, nan, 0.0038824844360351553, 0.0038824844360351553, nan, 0.0, 0.0, nan, 0.0, 0.0, nan, 0.0, 0.0, nan, 0.0, 0.0, nan, 0.0, 0.0, nan, 0.0, 0.0, nan, 0.0, 0.0, nan, 0.0, 0.0, nan, 0.0, 0.0, nan, 0.00019025802612304666, 0.00019025802612304666, nan, 0.0, 0.0, nan, 0.0, 0.0, nan, 0.0, 0.0, nan, 0.002421417236328125, 0.002421417236328125, nan, 0.0, 0.0, nan, 0.0006414413452148437, 0.0006414413452148437, nan, 0.007469778060913087, 0.007469778060913087, nan, 0.0, 0.0, nan, 0.0, 0.0, nan, 0.0, 0.0, nan, 0.0, 0.0, nan, 0.0, 0.0, nan, 0.0, 0.0, nan, 0.0, 0.0, nan, 0.0, 0.0, nan, 0.0156949234008789, 0.0156949234008789, nan, 0.026187481880187977, 0.026187481880187977, nan, 0.023743436932563776, 0.023743436932563776, nan, 0.028988721966743465, 0.028988721966743465, nan, 0.02145364582538604, 0.02145364582538604, nan, 0.011232057213783255, 0.011232057213783255, nan, 0.024074302315711966, 0.024074302315711966, nan, 0.0, 0.0, nan, 0.005289626121520995, 0.005289626121520995, nan, 0.025243592262268064, 0.025243592262268064, nan, 0.0072573709487915045, 0.0072573709487915045, nan, 0.0, 0.0, nan, 0.002139425277709961, 0.002139425277709961, nan, 0.0, 0.0, nan, 0.0, 0.0, nan, 0.0, 0.0, nan, 0.0, 0.0, nan, 0.0, 0.0, nan, 0.0, 0.0, nan, 0.0, 0.0, nan, 0.005034195780754091, 0.005034195780754091, nan, 0.0, 0.0, nan, 0.0, 0.0, nan, 0.011182727813720702, 0.011182727813720702, nan, 0.014443035125732414, 0.014443035125732414, nan, 0.03869737625122069, 0.03869737625122069, nan, 0.010358257293701132, 0.010358257293701132, nan, 0.0, 0.0, nan, 0.0, 0.0, nan, 0.0, 0.0, nan, 0.0, 0.0, nan, 0.0, 0.0, nan, 0.0, 0.0, nan, 0.0, 0.0, nan, 0.0, 0.0, nan, 0.0, 0.0, nan, 0.0, 0.0, nan, 0.0, 0.0, nan, 0.010822300016880039, 0.010822300016880039, nan, 0.0, 0.0, nan, 0.0, 0.0, nan, 0.0, 0.0, nan, 0.0, 0.0, nan, 0.0, 0.0, nan, 0.0, 0.0, nan, 0.0, 0.0, nan, 0.0, 0.0, nan, 0.0, 0.0, nan, 0.0, 0.0, nan, 0.0, 0.0, nan, 0.0, 0.0, nan, 0.0, 0.0, nan, 0.0, 0.0, nan, 0.0, 0.0, nan, 0.0, 0.0, nan, 0.0, 0.0, nan, 0.0, 0.0, nan, 0.0, 0.0, nan, 0.001330413818359375, 0.001330413818359375, nan, 0.0, 0.0, nan, 0.005959672927856445, 0.005959672927856445, nan, 0.0, 0.0, nan, 0.0, 0.0, nan, 0.007199201583862303, 0.007199201583862303, nan, 0.015323598384857178, 0.015323598384857178, nan, 0.006805078983306886, 0.006805078983306886, nan, 0.015063683986663825, 0.015063683986663825, nan, 0.0027363955974578887, 0.0027363955974578887, nan, 0.012695561647415168, 0.012695561647415168, nan, 0.014204474687576312, 0.014204474687576312, nan, 0.005719540715217604, 0.005719540715217604, nan, 0.01737168252468111, 0.01737168252468111, nan, 0.02141170442104342, 0.02141170442104342, nan, 0.017217719554901152, 0.017217719554901152, nan, 0.01012599721550945, 0.01012599721550945, nan, 0.01238225713372234, 0.01238225713372234, nan, 0.02997728124260906, 0.02997728124260906, nan, 0.0, 0.0, nan, 0.008400363922119142, 0.008400363922119142, nan, 0.01761590957641602, 0.01761590957641602, nan, 0.010009559690952293, 0.010009559690952293, nan, 0.008900764733552925, 0.008900764733552925, nan, 0.014991348534822459, 0.014991348534822459, nan, 0.009456551820039742, 0.009456551820039742, nan, 0.018010605126619325, 0.018010605126619325, nan, 0.011810782700777043, 0.011810782700777043, nan, 0.00289439991116523, 0.00289439991116523, nan, 0.023103605061769474, 0.023103605061769474]}, {[359.58929, 360.1004, 360.61145, 361.12241, 361.63336, 362.1442, 362.65503, 363.16577, 363.67648, 364.18713, 364.69769, 365.20825, 365.71872, 366.22913, 366.7395, 367.24979, 367.76004, 368.27023, 368.78036, 369.29047, 369.80051, 370.31049, 370.8204, 371.33026, 371.84009, 372.34985, 372.85956, 373.3692, 373.87881, 374.38834, 374.89786, 375.40729, 375.91669, 376.42599, 376.9353, 377.44452, 377.9537, 378.46283, 378.97192, 379.48093, 379.9899, 380.49881, 381.00769, 381.51651, 382.02527, 382.534, 383.04266, 383.55127, 384.05984, 384.56836, 385.07681, 385.58521, 386.09357, 386.6019, 387.11017, 387.61838, 388.12653, 388.63467, 389.14273, 389.65076, 390.15872, 389.65076, 390.15872, 390.66663, 391.17453, 391.68234, 392.19012, 392.69785, 393.20554, 393.71317, 394.22076, 394.7283, 395.23578, 395.74326, 396.25064, 396.758, 397.26532, 397.77258, 398.27979, 398.78696, 399.29407, 399.80115, 400.30817, 400.81516, 401.32211, 401.82901, 402.33585, 402.84265, 403.34943, 403.85614, 404.36282, 404.86945, 405.37604, 405.88257, 406.38907, 406.89554, 407.40195, 407.90833, 408.41464, 408.92093, 409.42715, 409.93335, 410.43951, 410.94562, 411.45169, 411.95773, 412.46371, 412.96964, 413.47556, 413.98141, 414.48724, 414.99301, 415.49875, 416.00446, 416.5101, 417.01572, 417.5213, 418.02682, 418.53235, 419.03778, 419.54321, 420.04858], [0.014012220551121871, 0.0, 0.0, 0.005994377136230469, 0.0, 0.0, 0.004224395751953125, 0.0, 0.0038824844360351553, 0.0, 0.0, 0.0, 0.0, 0.0, 0.0, 0.0, 0.0, 0.0, 0.00019025802612304666, 0.0, 0.0, 0.0, 0.002421417236328125, 0.0, 0.0006414413452148437, 0.007469778060913087, 0.0, 0.0, 0.0, 0.0, 0.0, 0.0, 0.0, 0.0, 0.0156949234008789, 0.026187481880187977, 0.023743436932563776, 0.028988721966743465, 0.02145364582538604, 0.011232057213783255, 0.024074302315711966, 0.0, 0.005289626121520995, 0.025243592262268064, 0.0072573709487915045, 0.0, 0.002139425277709961, 0.0, 0.0, 0.0, 0.0, 0.0, 0.0, 0.0, 0.005034195780754091, 0.0, 0.0, 0.011182727813720702, 0.014443035125732414, 0.03869737625122069, 0.010358257293701132, 0.0, 0.0, 0.0, 0.0, 0.0, 0.0, 0.0, 0.0, 0.0, 0.0, 0.0, 0.010822300016880039, 0.0, 0.0, 0.0, 0.0, 0.0, 0.0, 0.0, 0.0, 0.0, 0.0, 0.0, 0.0, 0.0, 0.0, 0.0, 0.0, 0.0, 0.0, 0.0, 0.001330413818359375, 0.0, 0.005959672927856445, 0.0, 0.0, 0.007199201583862303, 0.015323598384857178, 0.006805078983306886, 0.015063683986663825, 0.0027363955974578887, 0.012695561647415168, 0.014204474687576312, 0.005719540715217604, 0.01737168252468111, 0.02141170442104342, 0.017217719554901152, 0.01012599721550945, 0.01238225713372234, 0.02997728124260906, 0.0, 0.008400363922119142, 0.01761590957641602, 0.010009559690952293, 0.008900764733552925, 0.014991348534822459, 0.009456551820039742, 0.018010605126619325, 0.011810782700777043, 0.00289439991116523, 0.023103605061769474]}], 15 "All Input data in one Cluster":T1={"PAS amplitude"=[4.4502721e-10, 5.3865779e-10, 8.1175872e-10, 1.0442702e-09, 1.3361378e-09], "PAS amp Uncertainty"=[3.183917e-11, 2.9731387e-11, 4.6741631e-11, 5.8582465e-11, 9.6887734e-11], "Size parameters"=[1.4958234847930176, 1.6828014203921446, 1.8697793559912719, 2.056757291590399, 2.2437352271895263], "Number ofSizes"=5.0, "GeometricCrossSection"=[3.1415926535897934e-10, 3.9760782021995823e-10, 4.908738521234053e-10, 5.939573610693203e-10, 7.068583470577035e-10], "Wave Length"=420.04858, "SMPS Sizes"=[121.9, 126.3, 131.0, 135.8, 140.7, 145.9, 151.2, 156.8, 162.5, 168.5, 174.7, 181.1, 187.7, 194.6, 201.7, 209.1, 216.7, 224.7, 232.9, 241.4, 250.3, 259.5, 269.0, 278.8, 289.0, 299.6, 310.6, 322.0, 333.8, 346.0, 358.7, 371.8, 385.4, 399.5, 414.2, 429.4, 445.1, 461.4, 478.3, 495.8, 514.0, 532.8, 552.3], "Concentration"=[[0.0, 0.0, 0.0, 0.0, 0.0, 0.0, 0.0, 0.0, 0.0, 0.000594222, 0.0067148, 0.0325883, 0.0950329, 0.181348, 0.216099, 0.185692, 0.101524, 0.0383134, 0.00909043, 0.000780919, 0.0, 0.0, 0.000216077, 0.00198783, 0.0080372, 0.0204479, 0.0283157, 0.0335331, 0.022157, 0.0123005, 0.00284358, 0.000773561, 0.000252233, 0.000229051, 0.000520001, 0.000225684, 0.000138298, 0.000244182, 0.0, 0.0, 0.0, 0.0, 0.0], [0.0, 0.0, 0.0, 0.0, 0.0, 0.0, 0.0, 0.0, 0.0, 0.0, 0.0, 0.0, 0.000816489, 0.00845349, 0.0408459, 0.112602, 0.207837, 0.230678, 0.191195, 0.115028, 0.0385312, 0.00775818, 0.000694285, 0.0, 0.0, 5.45e-05, 0.000573695, 0.00252084, 0.00630844, 0.00962652, 0.0109084, 0.0108076, 0.0029388, 0.00150807, 0.000290999, 2.27e-05, 0.0, 0.0, 0.0, 0.0, 0.0, 0.0, 0.0], [0.0, 0.0, 0.0, 0.0, 0.0, 0.0, 0.0, 0.0, 0.0, 0.0, 0.0, 0.0, 0.0, 0.0, 0.0, 0.0010312, 0.010922, 0.0510087, 0.131879, 0.225192, 0.246535, 0.18825, 0.0982208, 0.0303467, 0.00671228, 0.000607538, 1.36e-05, 0.0, 0.0, 7.85e-05, 0.000394547, 0.00155356, 0.00182002, 0.00285395, 0.00143116, 0.000779854, 0.000340487, 0.0, 0.0, 0.0, 0.0, 0.0, 5.83e-05], [0.0, 0.0, 0.0, 0.0, 0.0, 0.0, 0.0, 0.0, 0.0, 0.0, 0.0, 0.0, 0.0, 0.0, 0.0, 0.0, 0.0, 0.0, 0.00139618, 0.0150043, 0.0584558, 0.144869, 0.242414, 0.233752, 0.174403, 0.0932754, 0.0278801, 0.00466978, 0.000461, 1.86e-05, 0.0, 0.0, 1.87e-05, 0.000141669, 0.000338039, 0.000948904, 0.00124014, 0.000405092, 0.0, 0.000308013, 0.0, 0.0, 0.0], [0.0, 0.0, 0.0, 0.0, 0.0, 0.0, 0.0, 0.0, 0.0, 0.0, 0.0, 0.0, 0.0, 0.0, 0.0, 0.0, 0.0, 0.0, 0.0, 0.0, 0.001984, 0.0181243, 0.0738336, 0.168822, 0.26219, 0.229236, 0.15382, 0.0682415, 0.0199068, 0.0034375, 0.000356967, 1.85e-05, 0.0, 0.0, 7.2e-06, 2.06e-05, 0.0, 0.0, 0.0, 0.0, 0.0, 0.0, 0.0]], "Double Charge Correction"=TRUE, "Extincation Factor"=1.0, "Diameter Factor"=1.0, "Diameter Offset"=0.0, "Extinction Factor Flag"=FALSE, "Diameter Factor Flag"=FALSE, "Diameter Offset Flag"=FALSE, "Sizes"=[], "ExtinctionOrAbsorptionOrScattering"=0, "Concentration(#/cc)"=[]} {"ExtinctionOrAbsorptionOrScattering" scale=0.0..2.0})   [LabVIEW 2013]
uses:
  ParticleDistributionData.ctl
  ReadBaesDataTypeDefinition.ctl
  GraphXYRefs.ctl
  GeneralDataForRIRetrieval.ctl
  RIandRIMCResults.ctl
  BaesDataTypeDefinition.ctl
  <vilib>/imath/engines/lvmath2/RunTimeEngine/NodeEndStatement/NIMS_NodeEndStatement_Output.vi
  <instcachedir>/0/NIMS_NodeEndStatement_Output_53EC0D466D134D7ABD903AC30B43404B.lvgen/NIMS_NodeEndStatement_Output_53EC0D466D134D7ABD903AC30B43404B_002.vi
  <vilib>/imath/engines/lvmath2/RunTimeEngine/ErrorHandling/NIMS_Finalize Error.vi
  <vilib>/imath/engines/lvmath2/RunTimeEngine/Managers/WorkSpace/UID Generator.vi
  <vilib>/imath/engines/lvmath2/RunTimeEngine/Managers/SymbolTable/Clear UID.vi
  <instcachedir>/0/NIMS_NodeEndStatement_Output_53EC0D466D134D7ABD903AC30B43404B.lvgen/NIMS_NodeEndStatement_Output_53EC0D466D134D7ABD903AC30B43404B_010.vi
  <vilib>/imath/engines/lvmath2/RunTimeEngine/RunTimeType/NIMS_RunTimeType_From StrictType (excl LVString).vi
  <instcachedir>/0/NIMS_RunTimeType_From StrictType (excl LVString)_4DEE718D6EB74582AA20236969C084FC.lvgen/NIMS_RunTimeType_From StrictType (excl LVString)_4DEE718D6EB74582AA20236969C084FC_000.vi
  <vilib>/imath/engines/lvmath2/RunTimeEngine/LocalVariableDefStatement/MC_LocalVariableDefStatement_Display.vi
  <vilib>/imath/engines/lvmath2/RunTimeEngine/Managers/SymbolTable/NIMS_WorkSpace.lvlib
panel:
  in  "Data type for All input data in one cluster":T1={"PAS amplitude"=[4.4502721e-10, 5.3865779e-10, 8.1175872e-10, 1.0442702e-09, 1.3361378e-09], "PAS amp Uncertainty"=[3.183917e-11, 2.9731387e-11, 4.6741631e-11, 5.8582465e-11, 9.6887734e-11], "Size parameters"=[1.4958234847930176, 1.6828014203921446, 1.8697793559912719, 2.056757291590399, 2.2437352271895263], "Number ofSizes"=5.0, "GeometricCrossSection"=[3.1415926535897934e-10, 3.9760782021995823e-10, 4.908738521234053e-10, 5.939573610693203e-10, 7.068583470577035e-10], "Wave Length"=420.04858, "SMPS Sizes"=[121.9, 126.3, 131.0, 135.8, 140.7, 145.9, 151.2, 156.8, 162.5, 168.5, 174.7, 181.1, 187.7, 194.6, 201.7, 209.1, 216.7, 224.7, 232.9, 241.4, 250.3, 259.5, 269.0, 278.8, 289.0, 299.6, 310.6, 322.0, 333.8, 346.0, 358.7, 371.8, 385.4, 399.5, 414.2, 429.4, 445.1, 461.4, 478.3, 495.8, 514.0, 532.8, 552.3], "Concentration"=[[0.0, 0.0, 0.0, 0.0, 0.0, 0.0, 0.0, 0.0, 0.0, 0.000594222, 0.0067148, 0.0325883, 0.0950329, 0.181348, 0.216099, 0.185692, 0.101524, 0.0383134, 0.00909043, 0.000780919, 0.0, 0.0, 0.000216077, 0.00198783, 0.0080372, 0.0204479, 0.0283157, 0.0335331, 0.022157, 0.0123005, 0.00284358, 0.000773561, 0.000252233, 0.000229051, 0.000520001, 0.000225684, 0.000138298, 0.000244182, 0.0, 0.0, 0.0, 0.0, 0.0], [0.0, 0.0, 0.0, 0.0, 0.0, 0.0, 0.0, 0.0, 0.0, 0.0, 0.0, 0.0, 0.000816489, 0.00845349, 0.0408459, 0.112602, 0.207837, 0.230678, 0.191195, 0.115028, 0.0385312, 0.00775818, 0.000694285, 0.0, 0.0, 5.45e-05, 0.000573695, 0.00252084, 0.00630844, 0.00962652, 0.0109084, 0.0108076, 0.0029388, 0.00150807, 0.000290999, 2.27e-05, 0.0, 0.0, 0.0, 0.0, 0.0, 0.0, 0.0], [0.0, 0.0, 0.0, 0.0, 0.0, 0.0, 0.0, 0.0, 0.0, 0.0, 0.0, 0.0, 0.0, 0.0, 0.0, 0.0010312, 0.010922, 0.0510087, 0.131879, 0.225192, 0.246535, 0.18825, 0.0982208, 0.0303467, 0.00671228, 0.000607538, 1.36e-05, 0.0, 0.0, 7.85e-05, 0.000394547, 0.00155356, 0.00182002, 0.00285395, 0.00143116, 0.000779854, 0.000340487, 0.0, 0.0, 0.0, 0.0, 0.0, 5.83e-05], [0.0, 0.0, 0.0, 0.0, 0.0, 0.0, 0.0, 0.0, 0.0, 0.0, 0.0, 0.0, 0.0, 0.0, 0.0, 0.0, 0.0, 0.0, 0.00139618, 0.0150043, 0.0584558, 0.144869, 0.242414, 0.233752, 0.174403, 0.0932754, 0.0278801, 0.00466978, 0.000461, 1.86e-05, 0.0, 0.0, 1.87e-05, 0.000141669, 0.000338039, 0.000948904, 0.00124014, 0.000405092, 0.0, 0.000308013, 0.0, 0.0, 0.0], [0.0, 0.0, 0.0, 0.0, 0.0, 0.0, 0.0, 0.0, 0.0, 0.0, 0.0, 0.0, 0.0, 0.0, 0.0, 0.0, 0.0, 0.0, 0.0, 0.0, 0.001984, 0.0181243, 0.0738336, 0.168822, 0.26219, 0.229236, 0.15382, 0.0682415, 0.0199068, 0.0034375, 0.000356967, 1.85e-05, 0.0, 0.0, 7.2e-06, 2.06e-05, 0.0, 0.0, 0.0, 0.0, 0.0, 0.0, 0.0]], "Double Charge Correction"=TRUE, "Extincation Factor"=1.0, "Diameter Factor"=1.0, "Diameter Offset"=0.0, "Extinction Factor Flag"=FALSE, "Diameter Factor Flag"=FALSE, "Diameter Offset Flag"=FALSE, "Sizes"=[], "ExtinctionOrAbsorptionOrScattering"=0, "Concentration(#/cc)"=[]} {"ExtinctionOrAbsorptionOrScattering" scale=0.0..2.0}
  out "GoodRIfit":i32=1
  in  "Threshold":dbl=3.0
  out "Multiple Charge correction Initiated":bool=TRUE
  out "error out":errorcluster
  out "Start Time Value":u32=79515247
  out "Elapsed Time (sec)":u32=87
  out "Normalized Residuals vs Size parameter":T7(graph)=[{"Size parameters"=[1.4958234847930176, 1.6828014203921446, 1.8697793559912719, 2.056757291590399, 2.2437352271895263], "Normalized Residuals"=[0.7931423359415002, 0.09713514831429684, -1.6472674938822935, 0.752549504344804, 0.10996106256996976]}]
  out "Number of Different Wavelengths":i32=122
  out "Loop Index":i32=121
  out "Extinction Graph":T8(graph)=[{"Ramp Pattern"=[1.4958234847930176, 1.6828014203921446, 1.8697793559912719, 2.056757291590399, 2.2437352271895263], "Extinction"=[4.4502721e-10, 5.3865779e-10, 8.1175872e-10, 1.0442702e-09, 1.3361378e-09]}, {"Ramp Pattern"=[1.4958234847930176, 1.6828014203921446, 1.8697793559912719, 2.056757291590399, 2.2437352271895263], "Extinction"=[4.70280190004678e-10, 5.415457517767005e-10, 7.347627400456595e-10, 1.0883564059982397e-09, 1.3467916865916122e-09]}, {"Ramp Pattern"=[1.4958234847930176, 1.4958234847930176, 1.4958234847930176, 1.6828014203921446, 1.6828014203921446, 1.6828014203921446, 1.8697793559912719, 1.8697793559912719, 1.8697793559912719, 2.056757291590399, 2.056757291590399, 2.056757291590399, 2.2437352271895263, 2.2437352271895263, 2.2437352271895263], "Extinction"=[nan, 4.7686638e-10, 4.1318804e-10, nan, 5.68389177e-10, 5.089264029999999e-10, nan, 8.585003509999999e-10, 7.65017089e-10, nan, 1.102852665e-09, 9.85687735e-10, nan, 1.433025534e-09, 1.239250066e-09]}]
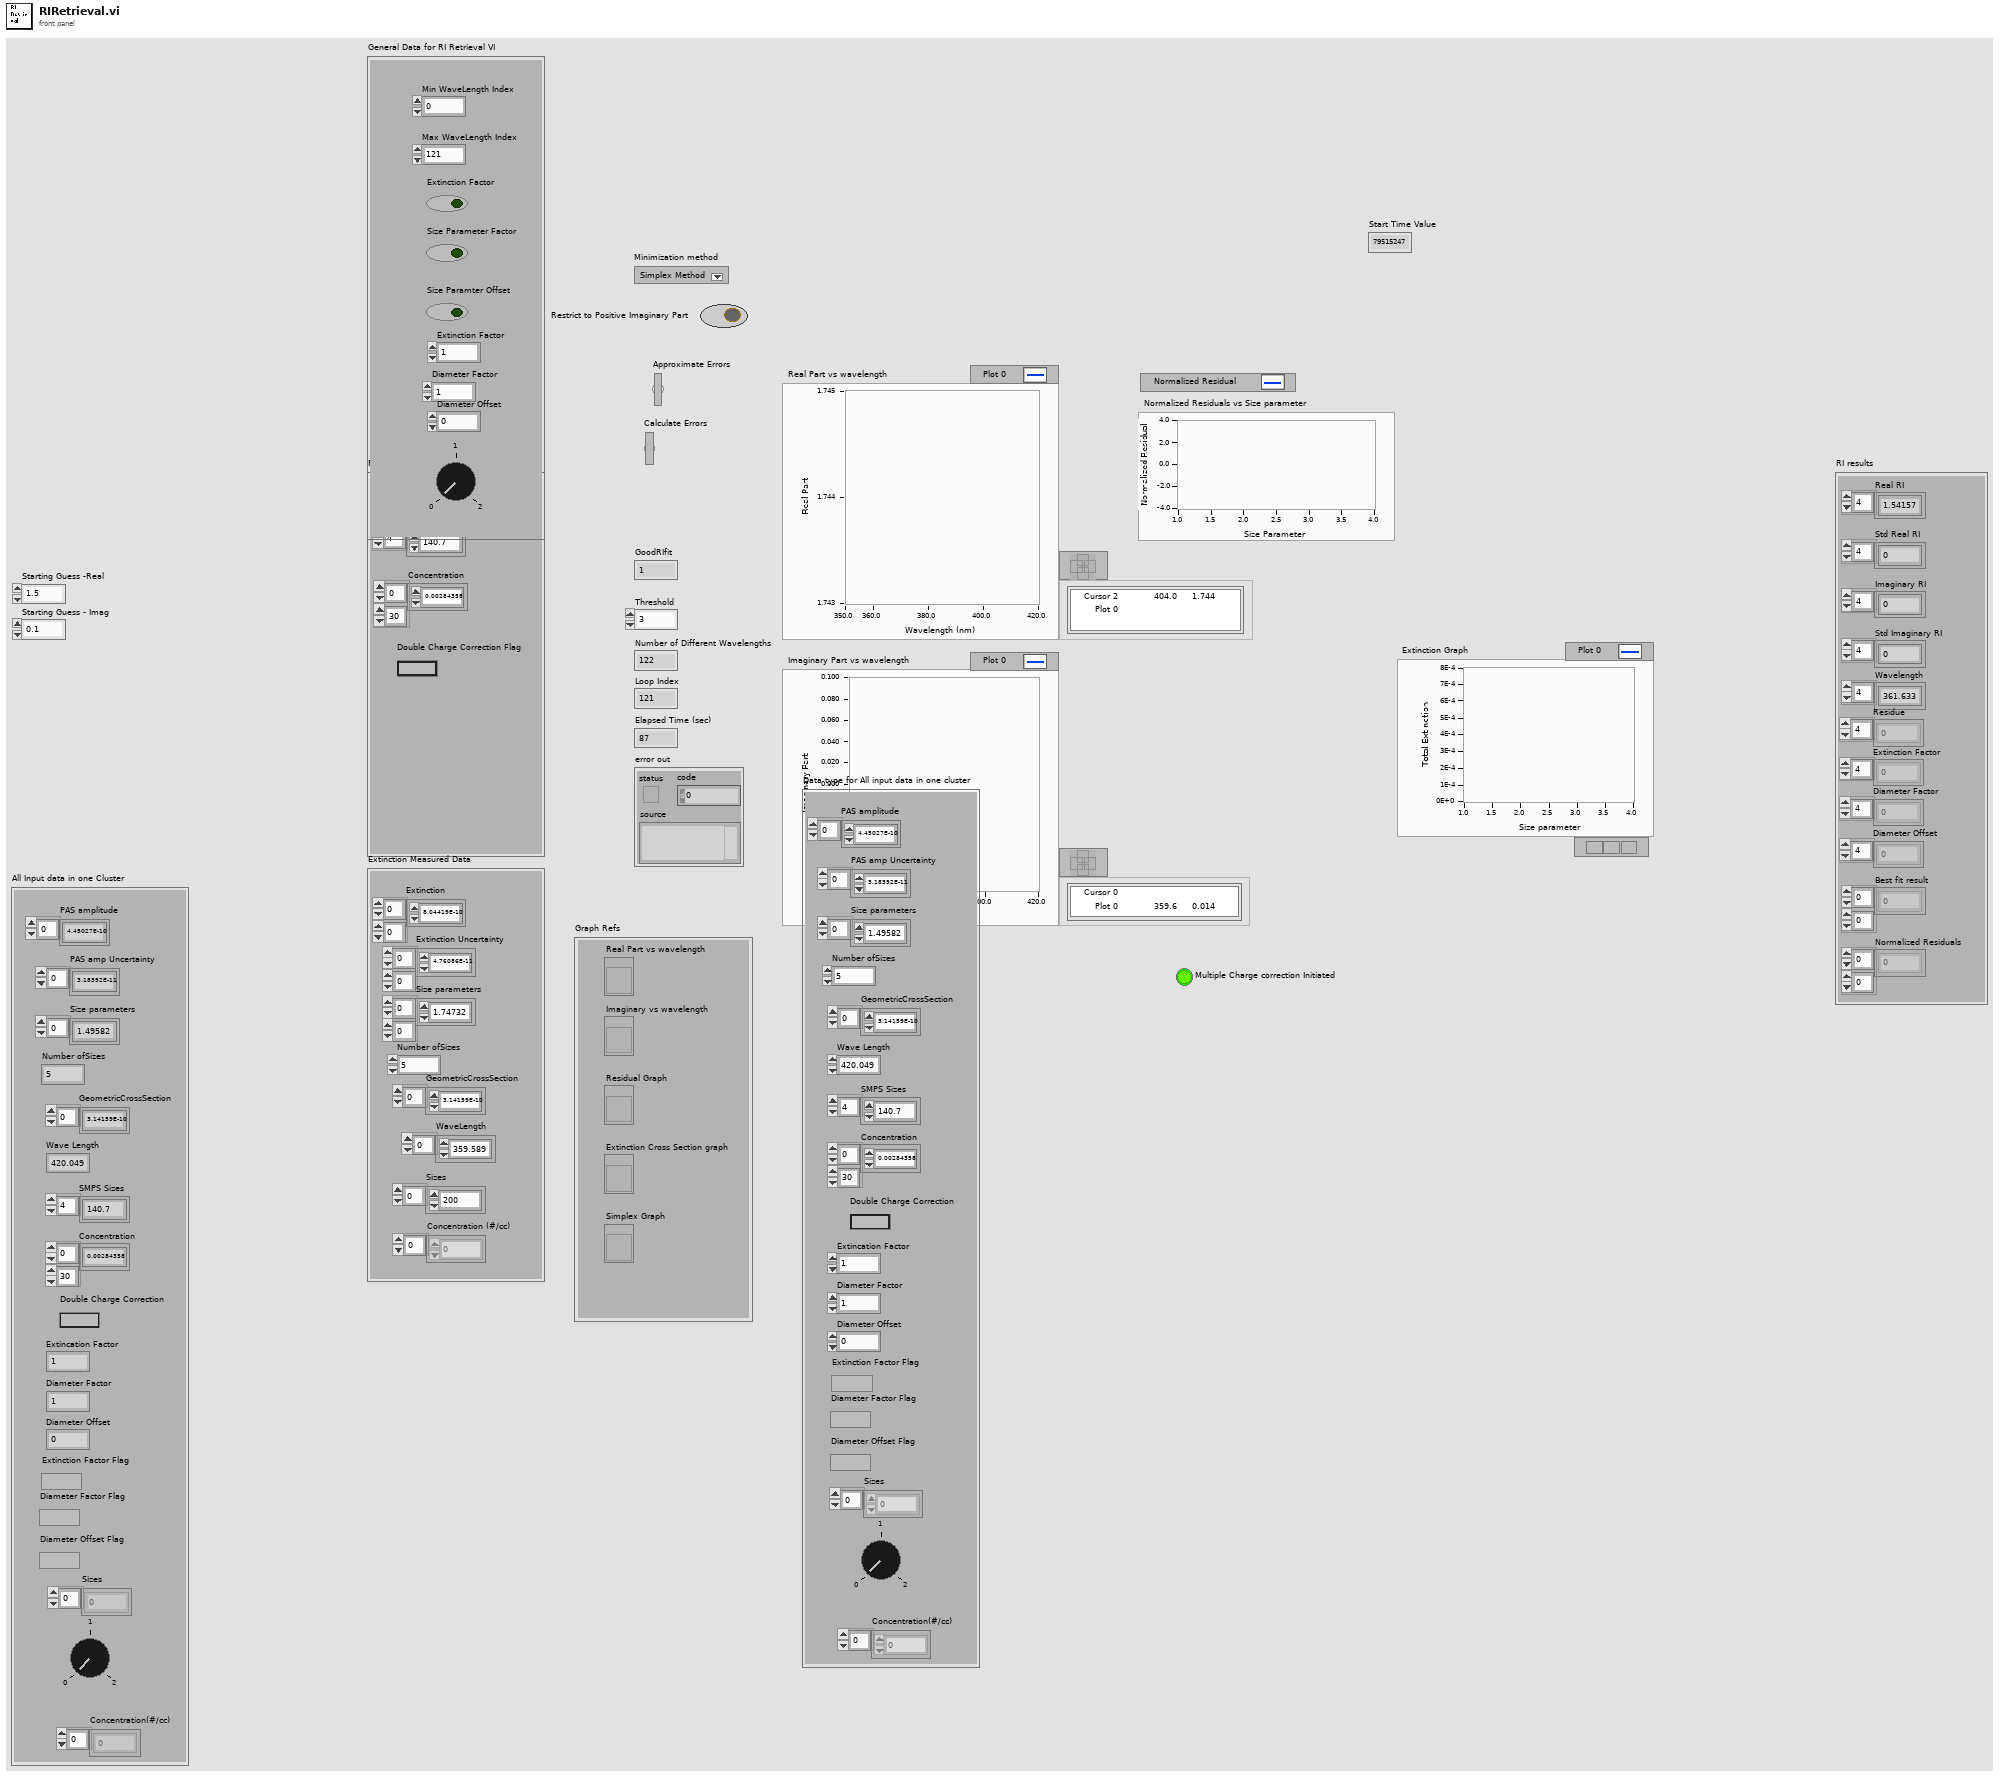
[diagram p1: front panel]
types:
  T1 = typedef "BaesDataTypeDefinition.ctl" = cluster{"PAS amplitude":dbl[], "PAS amp Uncertainty":dbl[], "Size parameters":dbl[], "Number ofSizes":dbl, "GeometricCrossSection":dbl[], "Wave Length":dbl, "SMPS Sizes":dbl[], "Concentration":dbl[][], "Double Charge Correction":bool, "Extincation Factor":dbl, "Diameter Factor":dbl, "Diameter Offset":dbl, "Extinction Factor Flag":bool, "Diameter Factor Flag":bool, "Diameter Offset Flag":bool, "Sizes":dbl[], "ExtinctionOrAbsorptionOrScattering":i8, "Concentration(#/cc)":dbl[]}
  T2 = typedef "RIandRIMCResults.ctl" = cluster{"Real RI":dbl[], "Imaginary RI":dbl[], "Std Imaginary RI":dbl[], "Std Real RI":dbl[], "Wavelength":dbl[], "Residue":dbl[], "Extinction Factor":dbl[], "Diameter Factor":dbl[], "Diameter Offset":dbl[], "Best fit result":dbl[][], "Normalized Residuals":dbl[][]}
  T3 = typedef "GeneralDataForRIRetrieval.ctl" = cluster{"Min WaveLength Index":u16, "Max WaveLength Index":u16, "Extinction Factor":bool, "Size Parameter Factor":bool, "Size Paramter Offset":bool, "Extinction Factor":dbl, "Diameter Factor":dbl, "Diameter Offset":dbl, "ExtinctionOrAbsorptionOrScattering":i8}
  T4 = typedef "GraphXYRefs.ctl" = cluster{"Real Part vs wavelength":refnum<vi>, "Imaginary vs wavelength":refnum<vi>, "Residual Graph":refnum<vi>, "Extinction Cross Section graph":refnum<vi>, "Simplex Graph":refnum<vi>}
  T5 = typedef "ReadBaesDataTypeDefinition.ctl" = cluster{"Extinction":dbl[][], "Extinction Uncertainty":dbl[][], "Size parameters":dbl[][], "Number ofSizes":dbl, "GeometricCrossSection":dbl[], "WaveLength":dbl[], "Sizes":dbl[], "Concentration (#/cc)":dbl[]}
  T6 = typedef "ParticleDistributionData.ctl" = cluster{"SMPS Sizes":dbl[], "Concentration":dbl[][], "Double Charge Correction Flag":bool}
  T7 = cluster{"Size parameters":dbl[], "Normalized Residuals":dbl[]}[]
  T8 = cluster{"Ramp Pattern":dbl[], "Extinction":dbl[]}[]
  T9 = cluster{"Size parameters":dbl[], "Extinction":dbl[]}[]
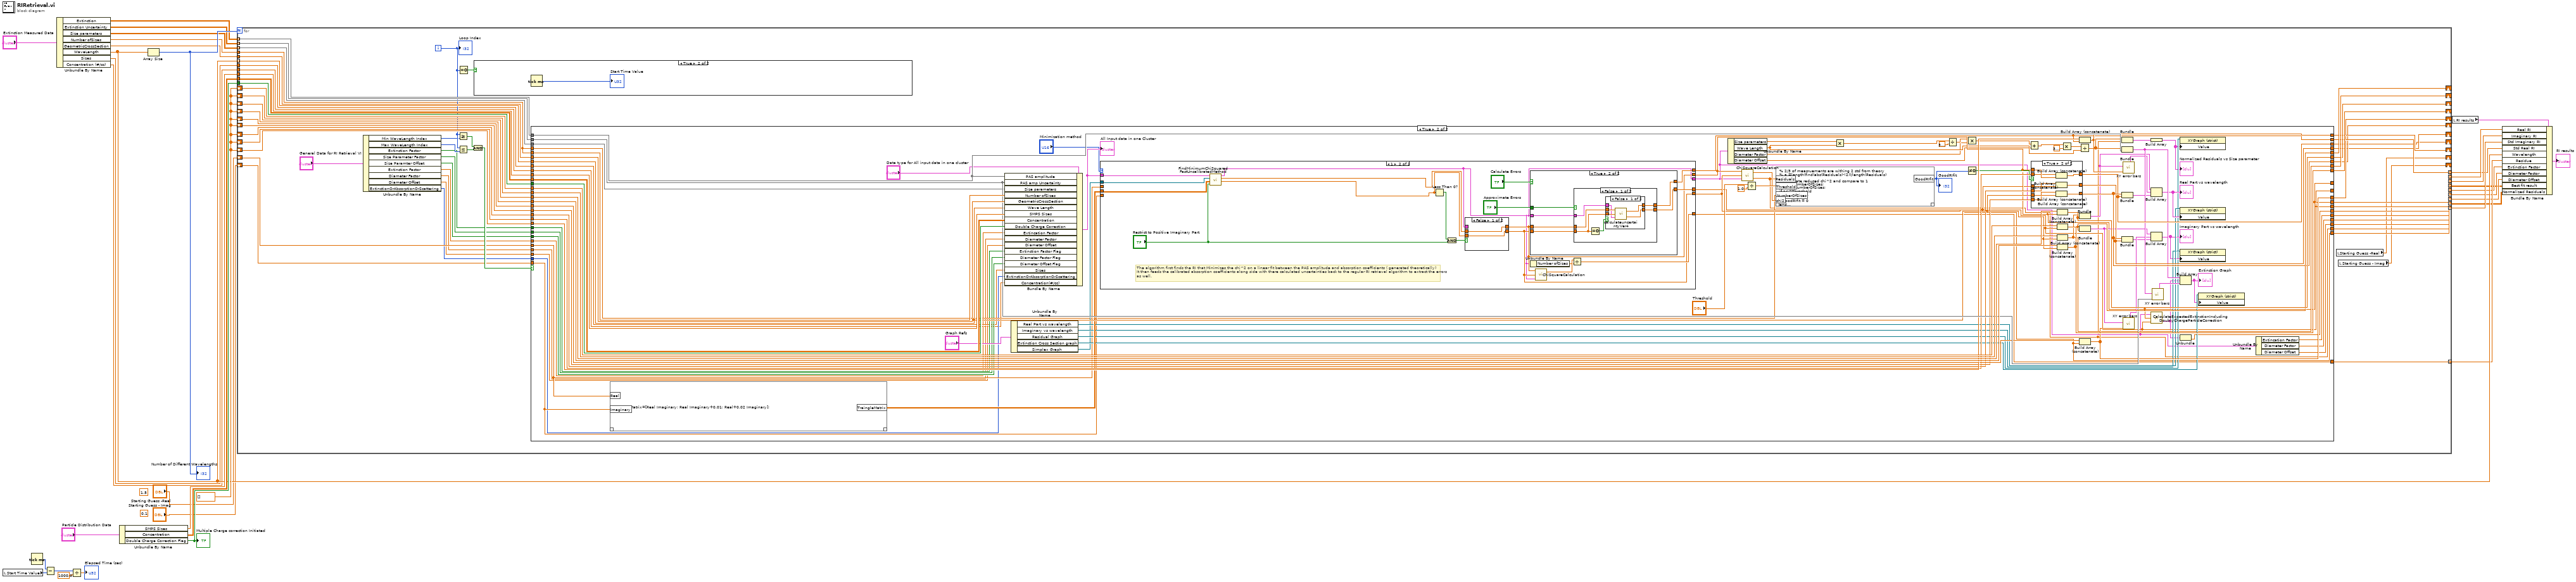
[diagram p0: block diagram]
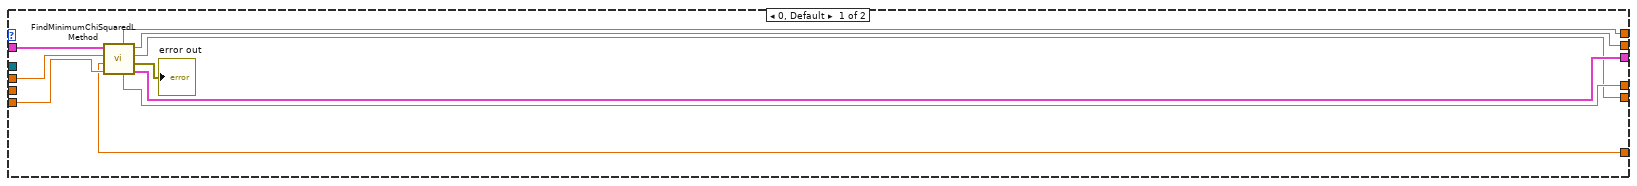
[diagram p4: hidden frame]
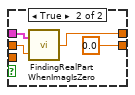
[diagram p5: hidden frame]
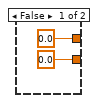
[diagram p6: hidden frame]
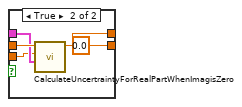
[diagram p7: hidden frame]
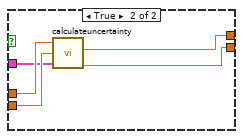
[diagram p8: hidden frame]
diagram:
  (unwired) 0.1 ("Imaginary Part from fit")
  (unwired) 1.5 ("Real Part from fit")
  w28 = dbl[] []
  n1 = local read "Start Time Value"() -> (w30:u32)
  n2 = Tick Count (ms)() -> (millisecond timer value=w34:u32)
  n3 = Subtract(x=w34, y=w30) -> (x-y=w32:u32)
  n4 = Unbundle By Name("Extinction Measured Data") -> ("Extinction"=w27:dbl[][], "Extinction Uncertainty"=w26:dbl[][], "Size parameters"=w25:dbl[][], "Number ofSizes"=w23:dbl, "GeometricCrossSection"=w24:dbl[], "WaveLength"=w11:dbl[], "Sizes"=w9:dbl[], "Concentration (#/cc)"=w3:dbl[])
  n5 = Divide(x=w32, y=1000.0) -> (x/y=→"Elapsed Time (sec)":dbl)
  n6 = Unbundle By Name("Particle Distribution Data") -> ("SMPS Sizes"=w20:dbl[], "Concentration"=w21:dbl[][], "Double Charge Correction Flag"=w22:bool)
  "Multiple Charge correction Initiated" <- w22
  n7 = Array Size(array=w11) -> (size(s)=w29:i32)
  "Number of Different Wavelengths" <- w29
  n8 = for {
    N: w29 -> [_]
    tunnel: [w67] -> w15 mode=indexing
    tunnel: [w69] -> w13 mode=indexing
    tunnel: [w78] -> w12 mode=indexing
    tunnel: [w76] -> w14 mode=indexing
    tunnel: w27 -> [w92] mode=indexing
    tunnel: w25 -> [w72] mode=indexing
    tunnel: w26 -> [w79] mode=indexing
    tunnel: w23 -> [w52]
    tunnel: w24 -> [w91]
    tunnel: w11 -> [w71] mode=indexing
    tunnel: w20 -> [w90]
    tunnel: w21 -> [w89]
    tunnel: w22 -> [w88]
    shift-right: [w84] -> _
    shift-left: w28 -> [w87]
    shift-right: [w85] -> _
    shift-left: w28 -> [w86]
    shift-right: [w83] -> _
    shift-left: w28 -> [w81]
    shift-right: [w82] -> _
    shift-left: w28 -> [w80]
    shift-right: [w74] -> _
    shift-left: w28 -> [w77]
    shift-right: [w73] -> _
    shift-left: w28 -> [w75]
    shift-right: [w63] -> _
    shift-left: w28 -> [w66]
    shift-right: [w64] -> _
    shift-left: w28 -> [w68]
    shift-right: [w65] -> _
    shift-left: w28 -> [w70]
    shift-right: [w36] -> _
    shift-left: "Starting Guess -Real" -> [w58]
    shift-right: [w35] -> _
    shift-left: "Starting Guess - Imag" -> [w57]
    tunnel: [w51] -> w10 mode=indexing
    tunnel: w9 -> [w47]
    tunnel: [w46] -> w8 mode=indexing
    tunnel: [w45] -> w7 mode=indexing
    tunnel: [w44] -> w6 mode=indexing
    tunnel: [w40] -> w5 mode=indexing
    tunnel: [w39] -> w4 mode=indexing
    tunnel: w3 -> [w37]
    i -> [w56]
    n9 = Unbundle By Name("General Data for RI Retrieval VI") -> ("Min WaveLength Index"=w54:u16, "Max WaveLength Index"=w53:u16, "Extinction Factor"=w50:bool, "Size Parameter Factor"=w49:bool, "Size Paramter Offset"=w48:bool, "Extinction Factor"=w42:dbl, "Diameter Factor"=w41:dbl, "Diameter Offset"=w43:dbl, "ExtinctionOrAbsorptionOrScattering"=w38:i8)
    n10 = Greater Or Equal?(x=w56, y=w54) -> (x >= y?=w60:bool)
    n11 = Less Or Equal?(x=w56, y=w53) -> (x <= y?=w59:bool)
    n12 = Equal To 0?(x=w56) -> (x = 0?=w62:bool)
    n13 = And(x=w60, y=w59) -> (x .and. y?=w61:bool)
    n14 = case shown="True" w62 {
      frame False {
      }
      frame True {
        n15 = Tick Count (ms)() -> (millisecond timer value=→"Start Time Value":u32)
      }
    }
    n16 = case shown="True" w61 {
      tunnel: w92 -> [_ w186]
      tunnel: w91 -> [_ w185]
      tunnel: w90 -> [_ w184]
      tunnel: w89 -> [_ w183]
      tunnel: w88 -> [_ w182]
      tunnel: w87 -> [_ w181]
      tunnel: w86 -> [_ w180]
      tunnel: w52 -> [_ w179]
      tunnel: [_ w136] -> w85
      tunnel: [_ w178] -> w84
      tunnel: [_ w177] -> w83
      tunnel: [_ w176] -> w82
      tunnel: w81 -> [_ w175]
      tunnel: w80 -> [_ w174]
      tunnel: w79 -> [_ w173]
      tunnel: [_ w130] -> w78
      tunnel: w77 -> [_ w172]
      tunnel: [_ w129] -> w76
      tunnel: w75 -> [_ w171]
      tunnel: [_ w170] -> w74
      tunnel: [_ w169] -> w73
      tunnel: w72 -> [_ w168]
      tunnel: w71 -> [_ w167]
      tunnel: w70 -> [_ w166]
      tunnel: [_ w133] -> w69
      tunnel: w68 -> [_ w165]
      tunnel: [_ w134] -> w67
      tunnel: w66 -> [_ w164]
      tunnel: [_ w163] -> w65
      tunnel: [_ w162] -> w64
      tunnel: [_ w161] -> w63
      tunnel: [w94 w134] -> _
      tunnel: [w93 w133] -> _
      tunnel: w58 -> [w94 w132]
      tunnel: w57 -> [w93 w131]
      tunnel: w52 -> [_ w127]
      tunnel: [_ w116] -> w51
      tunnel: w50 -> [_ w125]
      tunnel: w49 -> [_ w124]
      tunnel: w48 -> [_ w123]
      tunnel: w47 -> [_ w122]
      tunnel: [_ w120] -> w46
      tunnel: [_ w119] -> w45
      tunnel: [_ w118] -> w44
      tunnel: w43 -> [_ w102]
      tunnel: w42 -> [_ w101]
      tunnel: w41 -> [_ w100]
      tunnel: [_ w99] -> w40
      tunnel: [_ w97] -> w39
      tunnel: w38 -> [_ w96]
      tunnel: w37 -> [_ w95]
      frame False {
      }
      frame True {
        n17 = mathscript code="TraingleMatrix=[Real Imaginary; Real Imaginary+0.01; Real+0.02 Imaginary];"("Real"=w132, "Imaginary"=w131) -> ("TraingleMatrix"=w147:dbl[][])  [unwired: 1 in, 1 out]
        n18 = Bundle By Name(cluster="Data type for All input data in one cluster", "PAS amplitude"=w186, "PAS amp Uncertainty"=w173, "Size parameters"=w168, "Number ofSizes"=w179, "GeometricCrossSection"=w185, "Wave Length"=w167, "SMPS Sizes"=w184, "Concentration"=w183, "Double Charge Correction"=w182, "Extincation Factor"=w101, "Diameter Factor"=w100, "Diameter Offset"=w102, "Extinction Factor Flag"=w125, "Diameter Factor Flag"=w124, "Diameter Offset Flag"=w123, "Sizes"=w122, "ExtinctionOrAbsorptionOrScattering"=w96, "Concentration(#/cc)"=w95) -> (w121:T1)
        "All Input data in one Cluster" <- w121
        n19 = Unbundle By Name("Graph Refs") -> ("Real Part vs wavelength"=w144:refnum<vi>, "Imaginary vs wavelength"=w143:refnum<vi>, "Residual Graph"=w141:refnum<vi>, "Extinction Cross Section graph"=w138:refnum<vi>, "Simplex Graph"=w135:refnum<vi>)
        n20 = case shown="1" "Minimization method" {
          tunnel: [w306 w315] -> w134
          tunnel: [w297 w314] -> w133
          tunnel: w121 -> [w304 w310]
          tunnel: w147 -> [_ w312]
          tunnel: w135 -> [_ w313]
          tunnel: w132 -> [w303 _]
          tunnel: w131 -> [w302 _]
          tunnel: [w301 w320] -> w130
          tunnel: [w300 w319] -> w129
          tunnel: [w299 w316] -> w116
          tunnel: [w298 w309] -> w115
          frame 0, Default {
            n21 = call "FindMinimumChiSquaredLMethod.vi"("Extinction ExtinctionUncertainity Size parameter and Number ofS sizes 2"=w304, "Initial Guess for Real Part"=w303, "Initial Guess for Imaginary Part"=w302) -> ("residue"=w299:dbl, "Uncertainity in Real part"=w301:dbl, "Uncertainity in Imaginary part"=w300:dbl, "Real Part from fit"=w306:dbl, "Imaginary Part from fit"=w297:dbl, "error out"=→"error out":errorcluster, "Extinction ExtinctionUncertainity Size parameter and Number ofS sizes 3"=w298:T1)
          }
          frame 1 {
            # "The algorithm first finds the RI that Minimizes the chi^2 on a linear fit between the PAS amplitude and absorption coefficients ( generated theoretically)\nIt then feeds the calibrated absorption coefficients along side with there calculated uncertainties back to the regular RI retrieval algorithm to extract the errors\nas well."
            n22 = call "FindMinimumChiSquaredFastUncalibratedMethod.vi"("Restrict to Positive Imaginary Part"="Restrict to Positive Imaginary Part", "Starting points 2"=w312, "Simplex Graph"=w313, "Extinction ExtinctionUncertainity Size parameter and Number ofS sizes"=w310) -> ("Imaginary Part from fit"=w307:dbl, "Real Part from fit"=w308:dbl, "Extinction ExtinctionUncertainity Size parameter and Number ofS sizes 2"=w309:T1)  [unwired: 5 in]
            n23 = Less Than 0?(x=w307) -> (x < 0?=w322:bool)
            n24 = And(x=w322, y="Restrict to Positive Imaginary Part") -> (x .and. y?=w321:bool)
            n25 = case shown="False" w321 {
              tunnel: w308 -> [w326 w329]
              tunnel: w307 -> [w325 _]
              tunnel: [w326 w328] -> w315
              tunnel: [w325 0.0 ("Imaginary Part from fit")] -> w314
              tunnel: w309 -> [_ w327]
              frame False {
              }
              frame True {
                n26 = call "FindingRealPartWhenImagIsZero.vi"("Initial Guess Real"=w329, "Extinction ExtinctionUncertainity Size parameter and Number ofS sizes 2"=w327) -> ("Real"=w328:dbl)
              }
            }
            n27 = case shown="True" "Calculate Errors" {
              tunnel: w315 -> [_ w338]
              tunnel: w314 -> [_ w337]
              tunnel: [0.0 ("Uncertainty in Real part") w336] -> w320
              tunnel: [0.0 ("Uncertainty in Imaginary part") w335] -> w319
              tunnel: w309 -> [_ w334]
              tunnel: "Approximate Errors" -> [_ w333]
              frame False {
              }
              frame True {
                n28 = case shown="False" w333 {
                  tunnel: w338 -> [w344 w359]
                  tunnel: w337 -> [w339 w358]
                  tunnel: w334 -> [w343 w357]
                  tunnel: [w342 w356] -> w336
                  tunnel: [w341 w355] -> w335
                  frame False {
                    n29 = Equal To 0?(x=w339) -> (x = 0?=w340:bool)
                    n30 = case shown="False" w340 {
                      tunnel: w344 -> [w349 w354]
                      tunnel: w339 -> [w348 w352]
                      tunnel: w343 -> [w347 w353]
                      tunnel: [w346 w351] -> w342
                      tunnel: [w345 0.0 ("Uncertainty in Imaginary part")] -> w341
                      frame False {
                        n31 = call "calculateuncertaintyVer4.vi"("Extinction ExtinctionUncertainity Size parameter and Number ofS sizes 2"=w347, "refractive index, imaginary"=w348, "refractive index, real"=w349) -> ("Uncertainty in Imaginary part"=w345:dbl, "Uncertainty in Real part"=w346:dbl)
                      }
                      frame True {
                        n32 = call "CalculateUncertraintyForRealPartWhenImagisZero.vi"("Extinction ExtinctionUncertainity Size parameter and Number ofS sizes 2"=w353, "refractive index, imaginary"=w352, "refractive index, real"=w354) -> ("Uncertainty in the Real Part"=w351:dbl)  [unwired: 8 in]
                      }
                    }
                  }
                  frame True {
                    n33 = call "calculateuncertainty.vi"("refractive index, real"=w359, "refractive index, imaginary"=w358, "Extinction ExtinctionUncertainity Size parameter and Number ofS sizes 2"=w357) -> ("Uncertainty in Real part"=w356:dbl, "Uncertainty in Imaginary part"=w355:dbl)  [unwired: 2 out]
                  }
                }
              }
            }
            n34 = Unbundle By Name(w309) -> ("Number ofSizes"=w317:dbl)
            n35 = call "ChiSquareCalculation.vi"("Extinction ExtinctionUncertainity Size parameter and Number ofS sizes 2"=w309, "refractive index, imaginary"=w314, "refractive index, real"=w315) -> ("Chi Squared"=w318:dbl)  [unwired: 1 out]
            n36 = Divide(x=w318, y=w317) -> (x/y=w316:dbl)
          }
        }
        n37 = Unbundle By Name(w115) -> ("Size parameters"=w107:dbl[], "Wave Length"=w106:dbl, "Diameter Factor"=w105:dbl, "Diameter Offset"=w104:dbl)
        n38 = call "ChiSquareCalculation.vi"("Extinction ExtinctionUncertainity Size parameter and Number ofS sizes 2"=w115, "refractive index, imaginary"=w133, "refractive index, real"=w134) -> ("Normalized Residuals"=w99:dbl[], "Chi Squared"=w128:dbl)
        n39 = Divide(x="Threshold", y=1.0) -> (x/y=w152:dbl)
        n40 = mathscript code="% 2/3 of measruements are withing 2 std from theory\n% a =length(find(abs(Residuals)<2))/length(Residuals)\n\n% calculate reduced chi^2 and compare to 1\n%dof=NumberOfSizes;\na=chi2/NumberOfSizes;\nif a<=Threshold\n  GoodRIfit = 1\nelse \n  GoodRIfit = 0\nend\n%a=a*100;"("Residuals"=w99, "Threshold"=w152, "NumberOfSizes"=w127, "chi2"=w128) -> ("GoodRIfit"=w151:i32)  [unwired: 1 in, 1 out]
        "GoodRIfit" <- w151
        n41 = Multiply(x=w107, y=w106) -> (x*y=w114:dbl[])
        n42 = Divide(x=w114, y=3.141592653589793) -> (x/y=w112:dbl[])
        n43 = Multiply(x=w112, y=w105) -> (x*y=w111:dbl[])
        n44 = Not Equal To 0?(x=w151) -> (x != 0?=w150:bool)
        n45 = Add(x=w111, y=w104) -> (x+y=w110:dbl[])
        n46 = case shown="True" w150 {
          tunnel: w167 -> [_ w224]
          tunnel: [w215 w223] -> w163
          tunnel: w166 -> [w215 w222]
          tunnel: w133 -> [_ w221]
          tunnel: [w214 w220] -> w162
          tunnel: w165 -> [w214 w219]
          tunnel: w134 -> [_ w218]
          tunnel: [w213 w217] -> w161
          tunnel: w164 -> [w213 w216]
          frame False {
          }
          frame True {
            n47 = Build Array (concatenate)(w216, w218) -> (w217:dbl[])
            n48 = Build Array (concatenate)(w219, w221) -> (w220:dbl[])
            n49 = Build Array (concatenate)(w222, w224) -> (w223:dbl[])
          }
        }
        n50 = Build Array (concatenate)(w181, w134) -> (w178:dbl[])
        n51 = Build Array (concatenate)(w174, w133) -> (w176:dbl[])
        n52 = Build Array (concatenate)(w180, w167) -> (w136:dbl[])
        n53 = Build Array (concatenate)(w175, w167) -> (w177:dbl[])
        n54 = Multiply(x=w110, y=3.141592653589793) -> (x*y=w108:dbl[])
        n55 = Divide(x=w108, y=w106) -> (x/y=w103:dbl[])
        n56 = Build Array (concatenate)(w172, w130) -> (w170:dbl[])
        n57 = Bundle(w136, w178) -> (w158:cluster{dbl[], dbl[]})  [unwired: 1 in]
        n58 = Bundle(w177, w176) -> (w156:cluster{dbl[], dbl[]})  [unwired: 1 in]
        n59 = Build Array (concatenate)(w171, w129) -> (w169:dbl[])
        n60 = Bundle(w103, "Normalized Residuals"=w99) -> (w140:cluster{dbl[], "Normalized Residuals":dbl[]})  [unwired: 1 in]
        n61 = Bundle(w103, "Extinction"=w186) -> (w159:cluster{dbl[], "Extinction":dbl[]})  [unwired: 1 in]
        n62 = Bundle(w163, w161) -> (w149:cluster{dbl[], dbl[]})  [unwired: 1 in]
        n63 = Bundle(w163, w162) -> (w148:cluster{dbl[], dbl[]})  [unwired: 1 in]
        n64 = call "XY error bars.vi"("XY plot"=w158, "Yerror"=w170) -> ("Y error bars"=w157:cluster{dbl[], dbl[]})  [unwired: 6 in, 2 out]
        n65 = call "XY error bars.vi"("XY plot"=w156, "Yerror"=w169) -> ("Y error bars"=w155:cluster{dbl[], dbl[]})  [unwired: 6 in, 2 out]
        n66 = Build Array(w140) -> (w139:cluster{dbl[], "Normalized Residuals":dbl[]}[])
        "Normalized Residuals vs Size parameter" <- w139
        n67 = Build Array(w158, w157, w149) -> (w146:cluster{dbl[], dbl[]}[])
        "Real Part vs wavelength" <- w146
        n68 = Build Array(w156, w155, w148) -> (w142:cluster{dbl[], dbl[]}[])
        "Imaginary Part vs wavelength" <- w142
        n69 = call "CalculateExpectedExtinctionIncludingDoublyChargeParticleCorrection.vi"("refractive index, imaginary"=w133, "refractive index, real"=w134, "Extinction ExtinctionUncertainity Size parameter and Number ofS sizes"=w115) -> ("Expected Extinction graph"=w98:cluster{"Size parameters":dbl[], dbl[]})  [unwired: 1 out]
        n70 = call "XY error bars.vi"("XY plot"=w159, "Yerror"=w173) -> ("Y error bars"=w160:cluster{dbl[], dbl[]})  [unwired: 6 in, 2 out]
        n71 = property class="XYGraph (strict)"(reference=w141, "Value"=w139) -> ()  [unwired: 1 in, 2 out]
        n72 = property class="XYGraph (strict)"(reference=w144, "Value"=w146) -> ()  [unwired: 1 in, 2 out]
        n73 = property class="XYGraph (strict)"(reference=w143, "Value"=w142) -> ()  [unwired: 1 in, 2 out]
        n74 = Build Array(w159, w98, w160) -> (w137:T9)
        "Extinction Graph" <- w137
        n75 = Unbundle(w98) -> (w97:dbl[])  [unwired: 1 out]
        n76 = property class="XYGraph (strict)"(reference=w138, "Value"=w137) -> ()  [unwired: 1 in, 2 out]
        n77 = Unbundle By Name(w115) -> ("Extincation Factor"=w120:dbl, "Diameter Factor"=w119:dbl, "Diameter Offset"=w118:dbl)
      }
    }
    n78 = local read "Starting Guess -Real"() -> (w36:dbl)
    n79 = local read "Starting Guess - Imag"() -> (w35:dbl)
    "Loop Index" <- w56
  }
  n80 = local read "RI results"() -> (w16:T2)
  n81 = Bundle By Name(cluster=w16, "Real RI"=w15, "Imaginary RI"=w13, "Std Imaginary RI"=w14, "Std Real RI"=w12, "Wavelength"=w11, "Residue"=w10, "Extinction Factor"=w8, "Diameter Factor"=w7, "Diameter Offset"=w6, "Best fit result"=w4, "Normalized Residuals"=w5) -> (→"RI results":T2)
